vi "MegaAwesome_9_27_12a_JW.vi"() -> ()   [LabVIEW 2011]
uses:
  data/MegaAwesome_States.ctl
  <vilib>/Utility/inputDevices.llb/keyboardAcquire.vi
  <vilib>/Utility/file.llb/Read From Spreadsheet File (string).vi
  <vilib>/Utility/file.llb/Write To Spreadsheet File (string).vi
panel:
  out "Image Center X":i32
  in  "Disable Flag":bool
  out "Index":string
  in  "Slider Min":dbl=5.0
  in  "Slider Max":dbl=5.0
  out "Opj X Axis":string
  out "X Axis Display Type":string
  in  "Index-Sat":dbl=5.0
  in  "Index-Lin":dbl=5.0
  in  "IndexLog-Lin":dbl=5.0
  in  "IndexLog-Sat":dbl=5.0 caption="Num Pts"
  out "Lin Id-Log Used":dbl[](array[numeric])
  out "Lin-Vg Array-Log Used":dbl[](array[numeric])
  in  "New: Comments":string
  out "Save Array":string[][](array[string])
  out "Folder Index":i32 caption="Length"
  out "Sat Id-Used":dbl[](array[numeric])
  out "Sat Vg Array-Used":dbl[](array[numeric])
  out "Vg Array-Log-Used":dbl[](array[numeric])
  out "Sat Id-Log-Used":dbl[](array[numeric])
  out "Lin Id-Used":dbl[](array[numeric])
  out "Lin-Vg Array-Used":dbl[](array[numeric])
  out "Lin Vd":dbl
  out "Recorded Prop":T1
  out "Current State":T2
  in  "Main Tab Control":T3(tab)
  in  "Transfer File":path
  out "Transfer Folder":path
  in  "Transport\nFolder":path caption="Transport Folder"
  out "Transport\nFile":path caption="Transport File"
  in  "Image Folder":path
  out "Image File":path
  out "Fabrication Prop":T4
  out "Distances":i32[](array[numeric])
  in  "Zoom":i32(slide)=-3 scale=-5.0..5.0
  in  "Magnification":i32(ring) items=["5x", "10x", "20x", "50x", "80x"]
  in  "Undo Button":bool
  in  "Remove Button":bool
  in  "Transfer Plots":T5(tab)=enum."Saturation"
  in  "Lin-Trans Slider":dbl(slide) step=1.0 scale=-2.0..2.0 scale format="%#_1p"
  out "Sqrt-Lin":cluster{dbl[], dbl[]}[](graph)
  in  "Sat-Trans Slider":dbl(slide) step=1.0 scale=-2.0..2.0 scale format="%#_1p"
  out "Sqrt-Sat":cluster{dbl[], dbl[]}[](graph)
  out "Raw- Lin":cluster{dbl[], dbl[]}[](graph)
  out "Raw- Sat":cluster{dbl[], dbl[]}[](graph)
  in  "Log Plots":enum32{"Linear", "Saturation", "Transport"}(tab)=enum."Saturation"
  in  "Lin-Log Slider":dbl(slide) step=1.0 scale=-2.0..2.0 scale format="%#_1p"
  out "Lin-Log":cluster{dbl[], dbl[]}[](graph)
  in  "Sat-Log Slider":dbl(slide) step=1.0 scale=-2.0..2.0 scale format="%#_1p"
  out "Sat-Log":cluster{dbl[], dbl[]}[](graph)
  out "Transport":cluster{ext[], ext[]}[](graph)
  out "Transport Name:":string
  in  "Manual Controls":T6
  in  "File Controls":T7
  out "Date Recorded":string="Date Recorded" caption="Measured"
  out "Data Name:":string
  out "Image Name":string
  out "Date Created":string caption="Fabricated"
  in  "Comments:":string
  out "Rec: Length":dbl caption="Length" format="%#_3g"
  out "Rec: Width":dbl caption="Width" format="%#_4g"
  out "Rec: Dielectric (d)":dbl caption="Dielectric (d)" format="%#_3g"
  in  "New: Dielectric":dbl
  in  "New: Length":dbl
  in  "New: Width":dbl
  out "Rec: Temp":dbl caption="Sample Temp" format="%.1f"
  in  "New: Temp":dbl format="%.1f"
  out "Image Out":T8(plugin-control)
  in  "Num Pts":dbl=5.0
  in  "Num Pts Log":dbl=5.0 caption="Num Pts"
  out "Recorded Values Cluster":T9
  out "Calculated Values Cluster":T9 caption="Recorded Values Cluster"
  out "Re-Calculated Values Cluster":T9 caption="Recorded Values Cluster"
  in  "Independant Variable:":string(combo)="Length (um):"
  out "Image Preview":T8(plugin-control)
  out "Total Width":i32
  in  "Index Array":u16(ring) caption="Index" items=["1A", "1A", "1A", "1A", "1A", "1A", "1A", "1A", "1A", "1A", "1A", "1A", "1A", "1A", "1A", "1A", "1A", "1A", "1A", "1A", "1A", "1A", "1A", "1A", "1A", "1A", "1A", "1A", "1A", "1A", "1A", "1A", "1A", "1A", "1A", "1A", "1A"]
  in  "Room Temp":dbl=294.0 caption="Room Temp (K)"
  out "No Image\n File":path=path "\\\\acad1\\physics/Jurchescu-group/JW-PD/Mega Awesome/Image Not Found.png" caption="No Image File"
  out "Origin Project File":path=path "\\\\acad1\\physics/Jurchescu-group/JW-PD/Group Library/Origin Project Files/DeviceData_8_10_12a_JW.opj"
  out "No Transport\n File":path=path "\\\\acad1\\physics/Jurchescu-group/JW-PD/Mega Awesome/No Transport File.txt" caption="No Transport File"
  in  "Transport Style Controls":T10={"Transport Line Size"=1, "Transport Line Color"=16772608} {"Transport Line Size" items=["Extra Small", "Small", "Medium", "Large", "Extra Large"]}
  out "Application Directory":path
  # "1)  Select the Transfer File that you would like to analyze:"
  # "Transfer Location"
  # "2) What else would you like to view during your analysis?"
  # "Transport Location"
  # "Image Location"
  # "Recorded"
  # "Calculated"
  # "Re-Calculated"
  # "Manual"
  # "um"
  # "Slider\nDoesn't\nWork"
  # "V"
  # "V"
  # "Slider\nDoesn't\nWork"
  # "V"
  # "Default File Choices"
  # "Default Analysis Values"
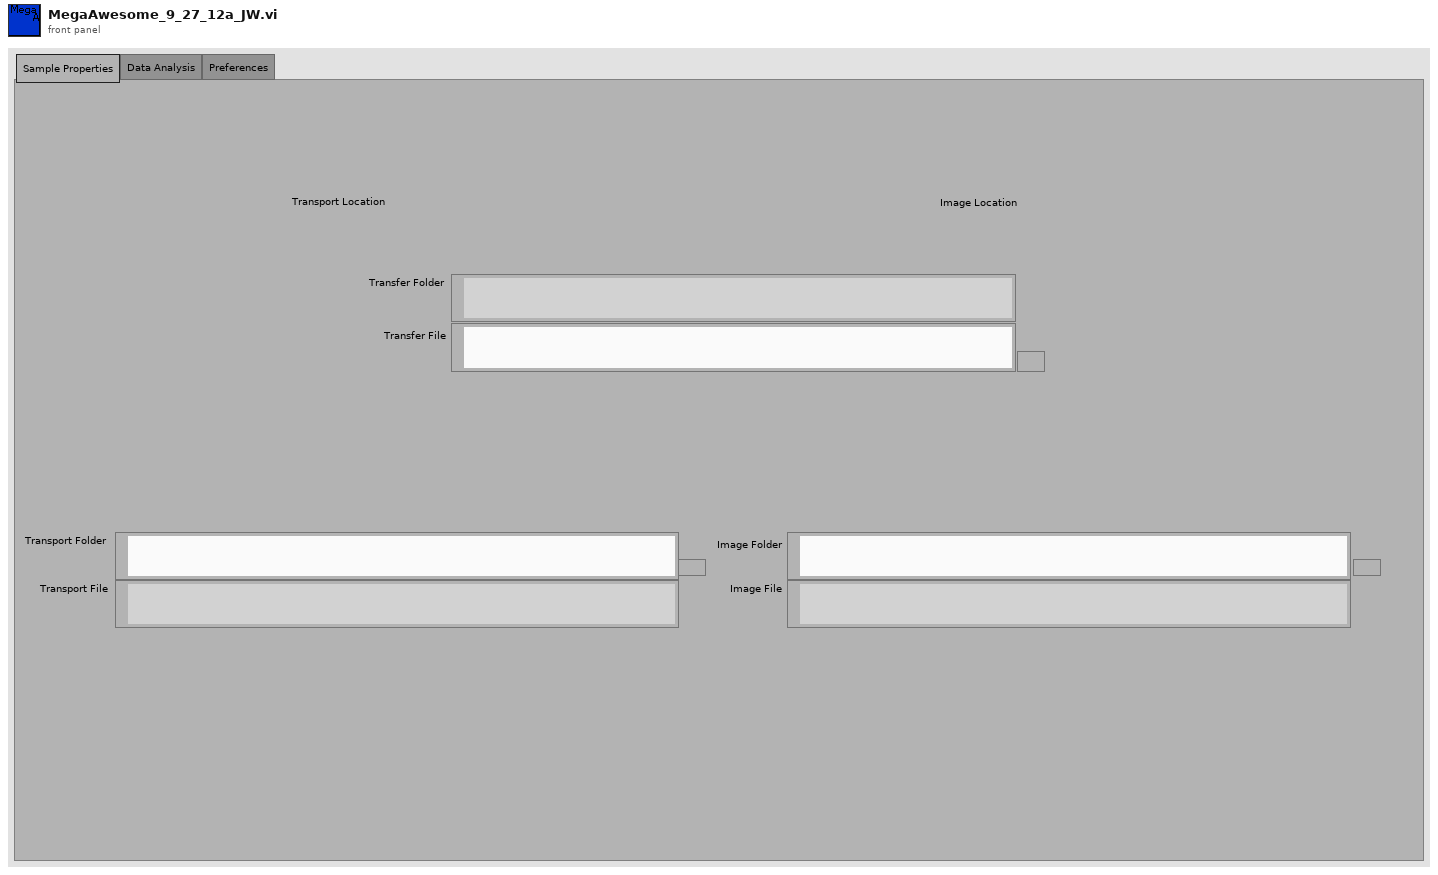
[diagram p1: front panel]
types:
  T1 = cluster{"Date Recorded":string, "Index":string, "Length":dbl, "Width":dbl, "Sample Temp":dbl}
  T2 = typedef "MegaAwesome_States.ctl" = enum16{"Init", "File Missing", "No Event", "Read Data", "Calculated Values", "Re-Calculated Values", "Next File", "Previous File", "Discard File", "Save", "Save Lines", "Export", "Exit"}
  T3 = enum32{"Sample Properties", "Data Analysis", "Preferences"}
  T4 = cluster{"Date Created":string, "Material":string, "Solvent":string, "Concentration":dbl, "Method":string, "Dielectric (nm)":dbl, "Treatment":string, "Comments":string}
  T5 = enum32{"Linear", "Saturation", "Raw-Linear", "Raw-Saturation"}
  T6 = cluster{"Manual-Temp":bool, "Manual-Width":bool, "Manuel-Length":bool, "Manuel-Dielectric":bool, "Manual Comments":bool}
  T7 = cluster{"Previous File":bool, "Discard ":bool, "Save Lines":bool, "Close":bool, "Next File ":bool, "Save":bool, "Save Next":bool, "Export":bool}
  T8 = typedef "IMAQ Image.ctl" = refnum<image>
  T9 = cluster{"Mobility-Sat":dbl, "Moblitity-Lin":dbl, "On/Off":dbl, "Off Current":dbl, "Vt-Sat":dbl, "STS":dbl, "Trap Density-VT":dbl, "Trap Density-STS":dbl}
  T10 = cluster{"Transport Line Size":u16, "Transport Line Color":u32}
  T11 = typedef "LVBoundsTypeDef.ctl" = cluster{"Width":u32, "Height":u32}
  T12 = enum16{"0", "1", "2", "3", "4", "5", "6", "7", "8", "9", "A", "B", "C", "D", "E", "F", "G", "H", "I", "J", "K", "L", "M", "N", "O", "P", "Q", "R", "S", "T", "U", "V", "W", "X", "Y", "Z", "F1", "F2", "F3", "F4", "F5", "F6", "F7", "F8", "F9", "F10", "F11", "F12", "F13", "F14", "F15", "ADD", "BACK", "BACKSLASH", "CAPITAL", "COMMA", "DECIMAL", "DELETE", "DIVIDE", "DOWN", "END", "EQUALS", "ESCAPE", "GRAVE (`)", "HOME", "INSERT", "LBRACKET", "LCONTROL", "LEFT", "L ALT", "LSHIFT", "LWIN", "MINUS", "MULTIPLY", "NEXT", "NUMLOCK", "NUMPAD_0", "NUMPAD_1", "NUMPAD_2", "NUMPAD_3", "NUMPAD_4", "NUMPAD_5", "NUMPAD_6", "NUMPAD_7", "NUMPAD_8", "NUMPAD_9", "PAUSE", "PERIOD", "PRIOR (PG UP)", "RBRACKET", "RCONTROL", "RETURN", "RIGHT", "R ALT", "RSHIFT", "RWIN", "SCROLL", "SEMICOLON", "SLASH", "SPACE", "SUBTRACT", "TAB", "UP", "ENTER (num pad)", "' (quote)"}[]
  T13 = enum16{"0", "1", "2", "3", "4", "5", "6", "7", "8", "9", "A", "B", "C", "D", "E", "F", "G", "H", "I", "J", "K", "L", "M", "N", "O", "P", "Q", "R", "S", "T", "U", "V", "W", "X", "Y", "Z", "F1", "F2", "F3", "F4", "F5", "F6", "F7", "F8", "F9", "F10", "F11", "F12", "F13", "F14", "F15", "ADD", "BACK", "BACKSLASH", "CAPITAL", "COMMA", "DECIMAL", "DELETE", "DIVIDE", "DOWN", "END", "EQUALS", "ESCAPE", "GRAVE (`)", "HOME", "INSERT", "LBRACKET", "LCONTROL", "LEFT", "L ALT", "LSHIFT", "LWIN", "MINUS", "MULTIPLY", "NEXT", "NUMLOCK", "NUMPAD_0", "NUMPAD_1", "NUMPAD_2", "NUMPAD_3", "NUMPAD_4", "NUMPAD_5", "NUMPAD_6", "NUMPAD_7", "NUMPAD_8", "NUMPAD_9", "PAUSE", "PERIOD", "PRIOR (PG UP)", "RBRACKET", "RCONTROL", "RETURN", "RIGHT", "R ALT", "RSHIFT", "RWIN", "SCROLL", "SEMICOLON", "SLASH", "SPACE", "SUBTRACT", "TAB", "UP", "ENTER (num pad)", "' (quote)"}
  T14 = typedef "ROI Descriptor" = cluster{"Global Rectangle":i32[], "Contours":cluster{"ID":enum32{"External", "Internal"}, "Type":u32, "Coordinates":i32[]}[]}
  T15 = cluster{string, sgl, bool, bool, bool, bool, bool, bool, i32}
  T16 = cluster{i32, cluster{string, sgl, bool, bool, bool, bool, bool, bool, i32}, i32, i32}
  T17 = cluster{"Global Rectangle":i32[], "Contours":cluster{"Contour Type":u32, "ROI Type":u32, "Points":i32[]}[]}
  T18 = cluster{"Contour Type":u32, "ROI Type":u32, "Points":i32[]}[]
  T19 = cluster{"[0]":cluster{dbl[], dbl[]}, "[1]":cluster{dbl[], dbl[]}, "[2]":cluster{dbl[], dbl[]}, "[3]":cluster{dbl[], dbl[]}, "[4]":cluster{dbl[], dbl[]}, "[5]":cluster{dbl[], dbl[]}, "[6]":cluster{dbl[], dbl[]}, "[7]":cluster{dbl[], dbl[]}, "[8]":cluster{dbl[], dbl[]}}
  T20 = cluster{i32[], cluster{"Contour Type":u32, "ROI Type":u32, "Points":i32[]}[]}
  T21 = cluster{"Contour Type":u32, "ROI Type":u32, "Points":i32[]}
  T22 = cluster{"Points[0]":i32, "Points[1]":i32, "Points[2]":i32, "Points[3]":i32, "Points[4]":i32, "Points[5]":i32, "Points[6]":i32, "Points[7]":i32, "Points[8]":i32}
  T23 = cluster{"Sat Vg Used":dbl[], "Sat Sqrt(Id) Used ":dbl[], "Lin Vg Used":dbl[], "Lin Sqrt(Id) Used":dbl[], "Index-Lin":dbl, "Index-Sat":dbl}
  T24 = cluster{"Raw Sat":cluster{dbl[], dbl[]}[], "Sqrt Sat":cluster{dbl[], dbl[]}[], "Log Sat":cluster{dbl[], dbl[]}[], "Raw Lin":cluster{dbl[], dbl[]}[], "Sqrt Lin":cluster{dbl[], dbl[]}[], "Log Lin":cluster{dbl[], dbl[]}[]}
  T25 = cluster{"Mobility-Sat":dbl, "Vt-Sat":dbl, "Mobility-Lin":dbl, "Vt-Lin":dbl, "Off I-Sat":dbl, "On/Off I-Sat":dbl}
  T26 = cluster{"Sat Vg Used":dbl[], "Sat Log(Id) Used":dbl[], "Lin Vg Used":dbl[], "Lin Log(Id) Used":dbl[], "STS Index-Sat":dbl, "STS Index-Lin":dbl}
  T27 = cluster{"Independant  Variable Indicator":string, "Parameter String Indicator":string}
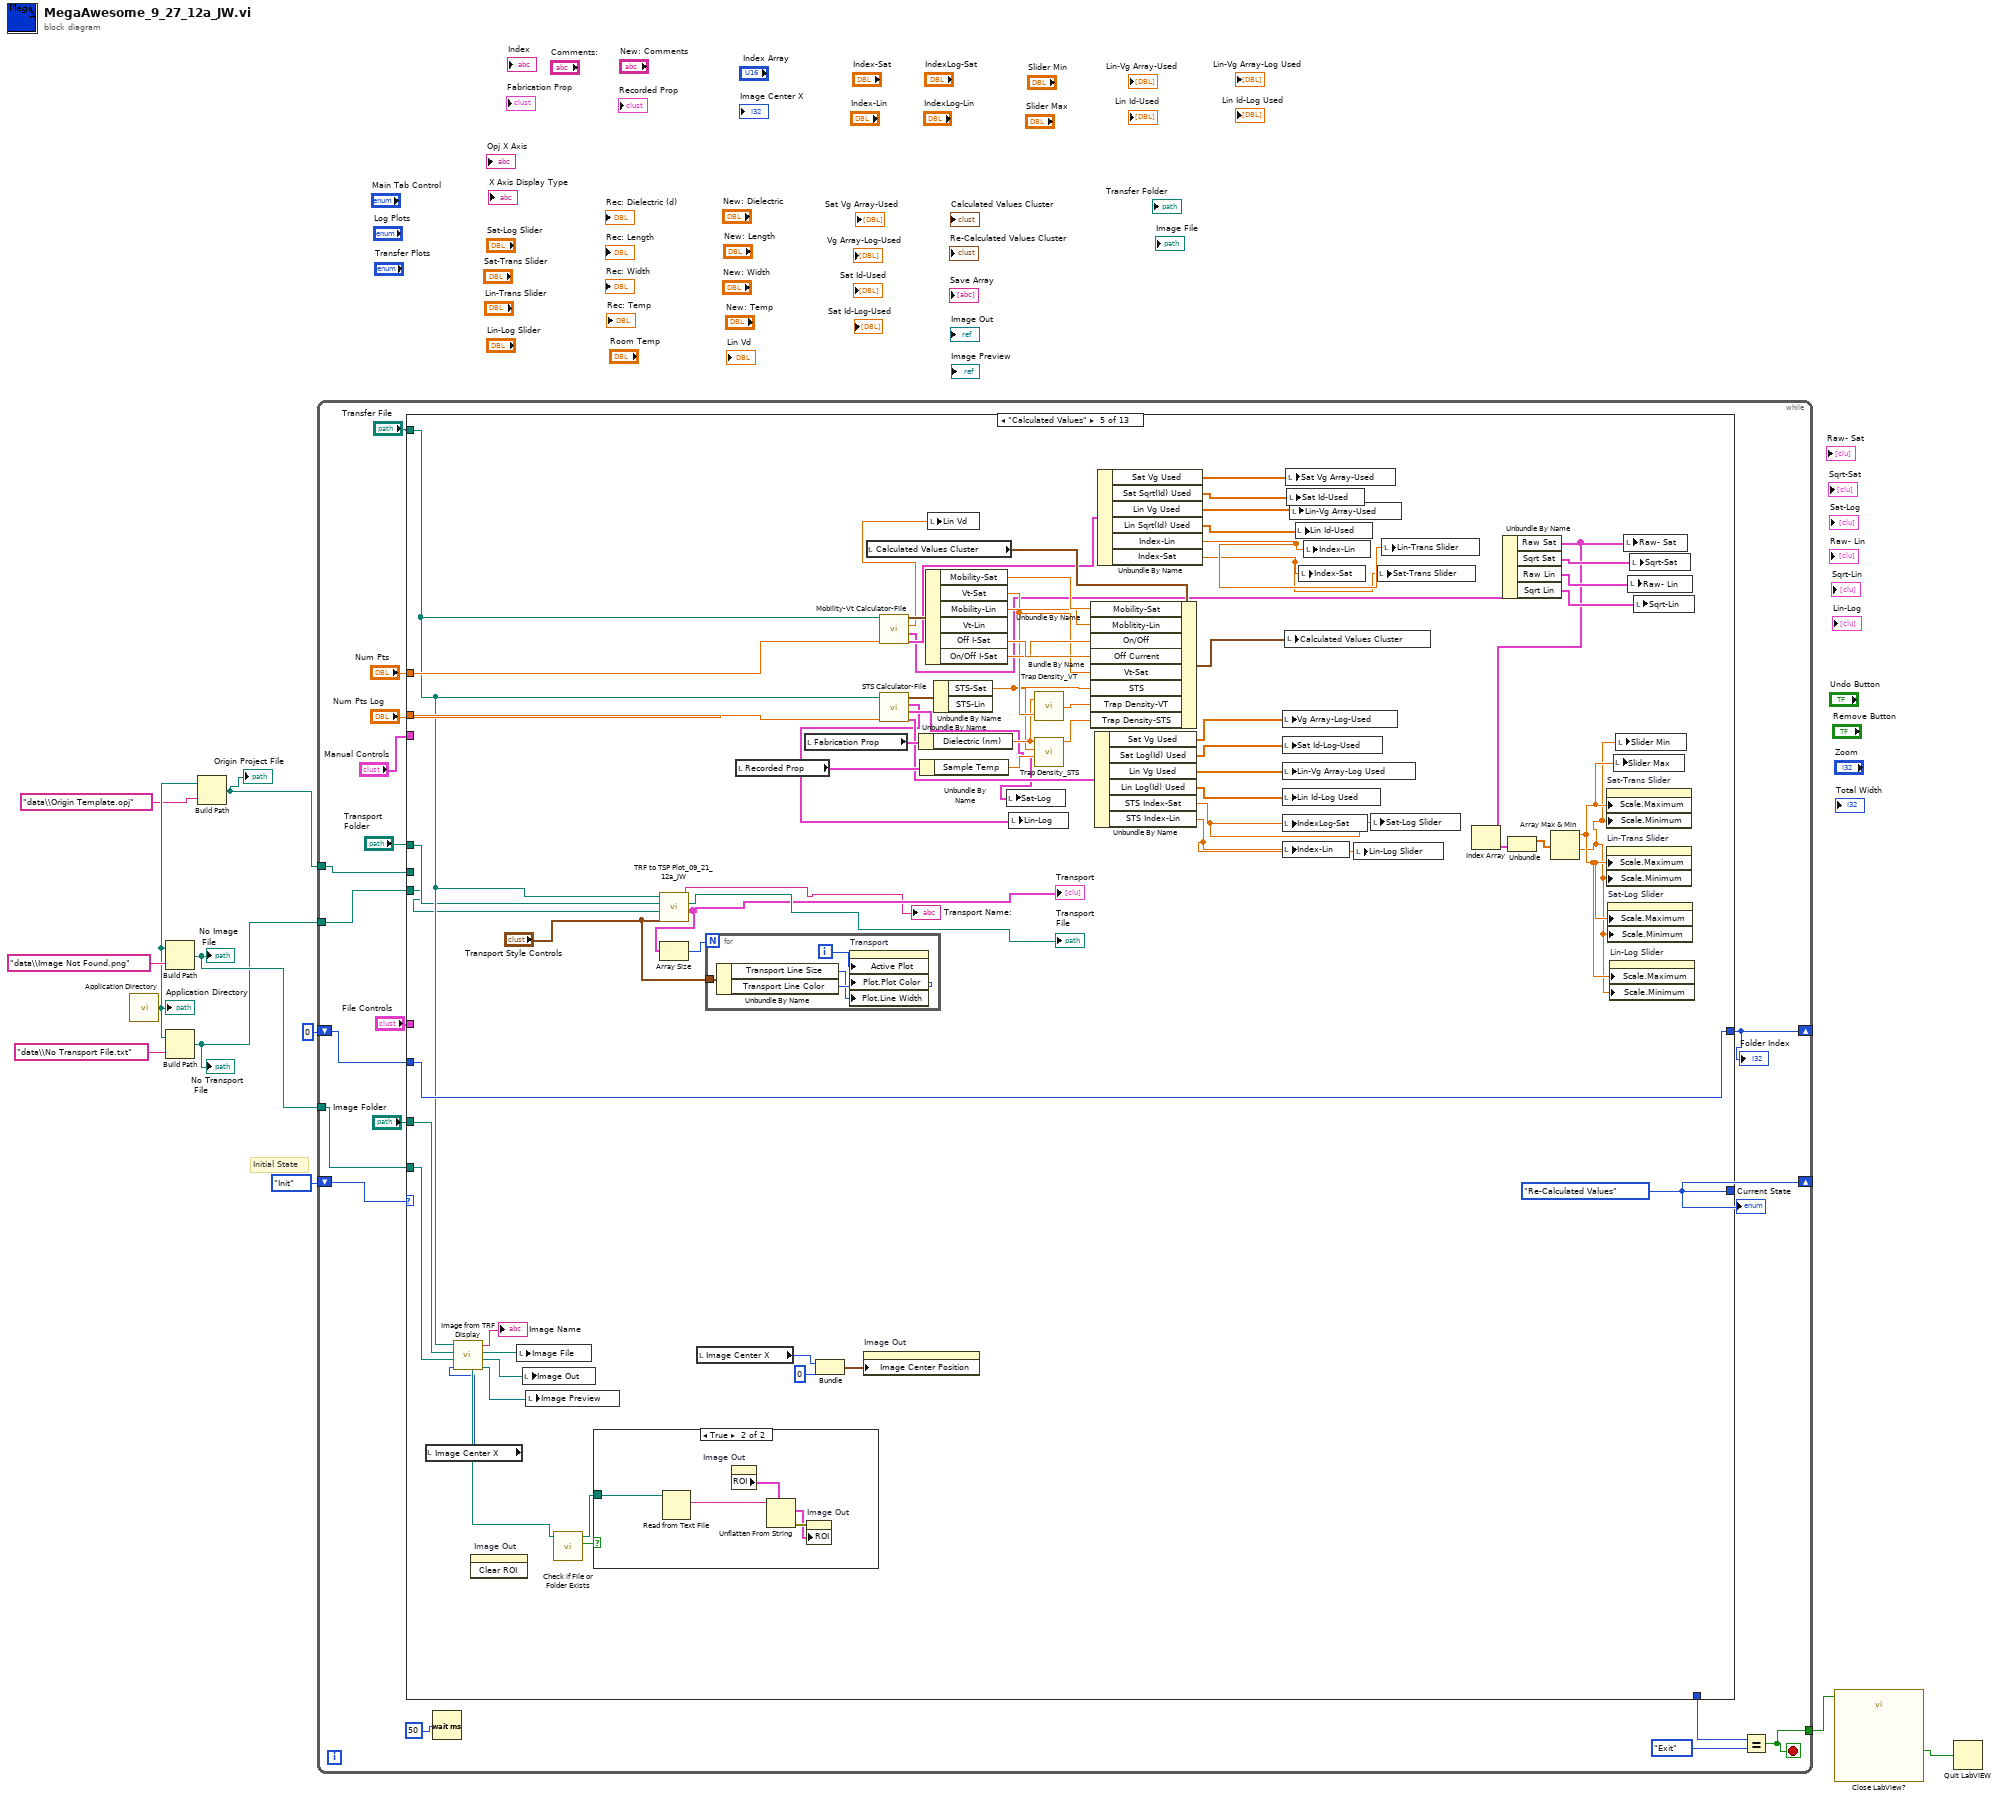
[diagram p0: block diagram]
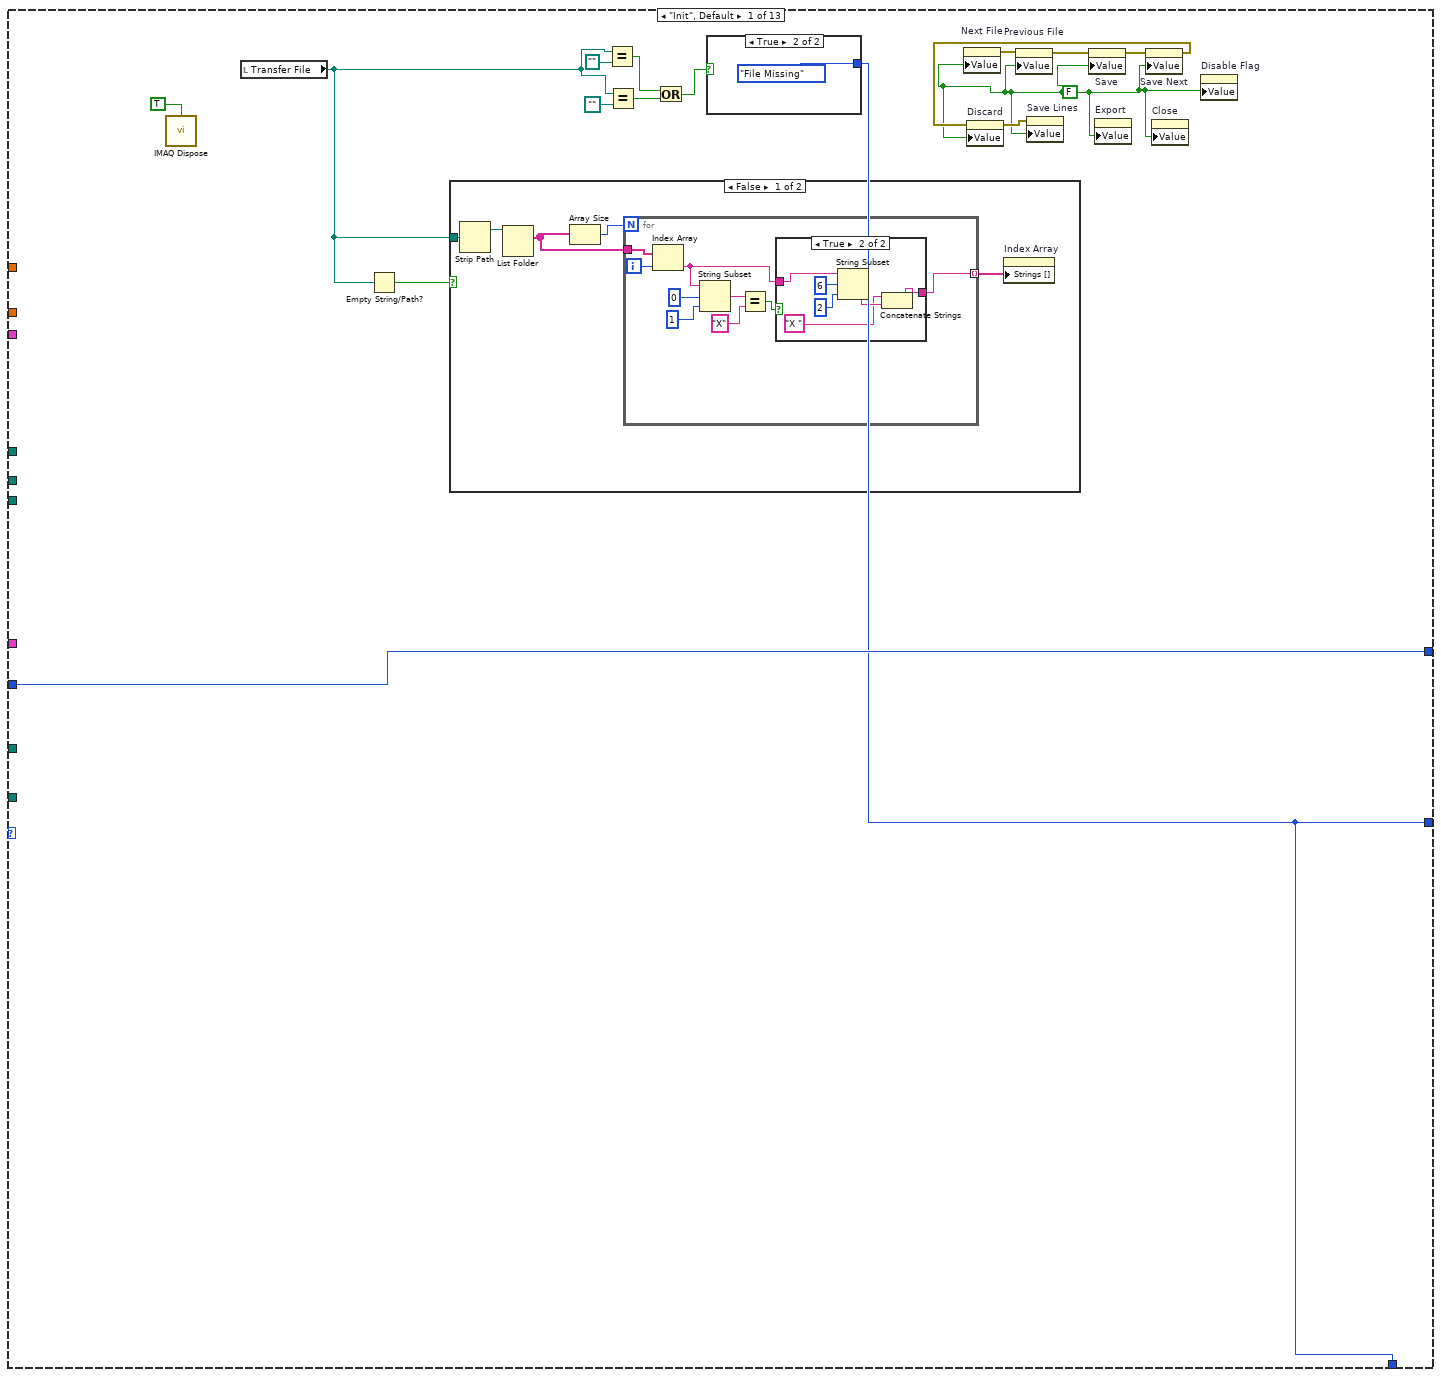
[diagram p2: hidden frame]
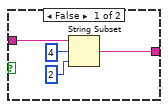
[diagram p3: hidden frame]
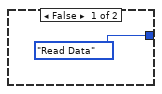
[diagram p5: hidden frame]
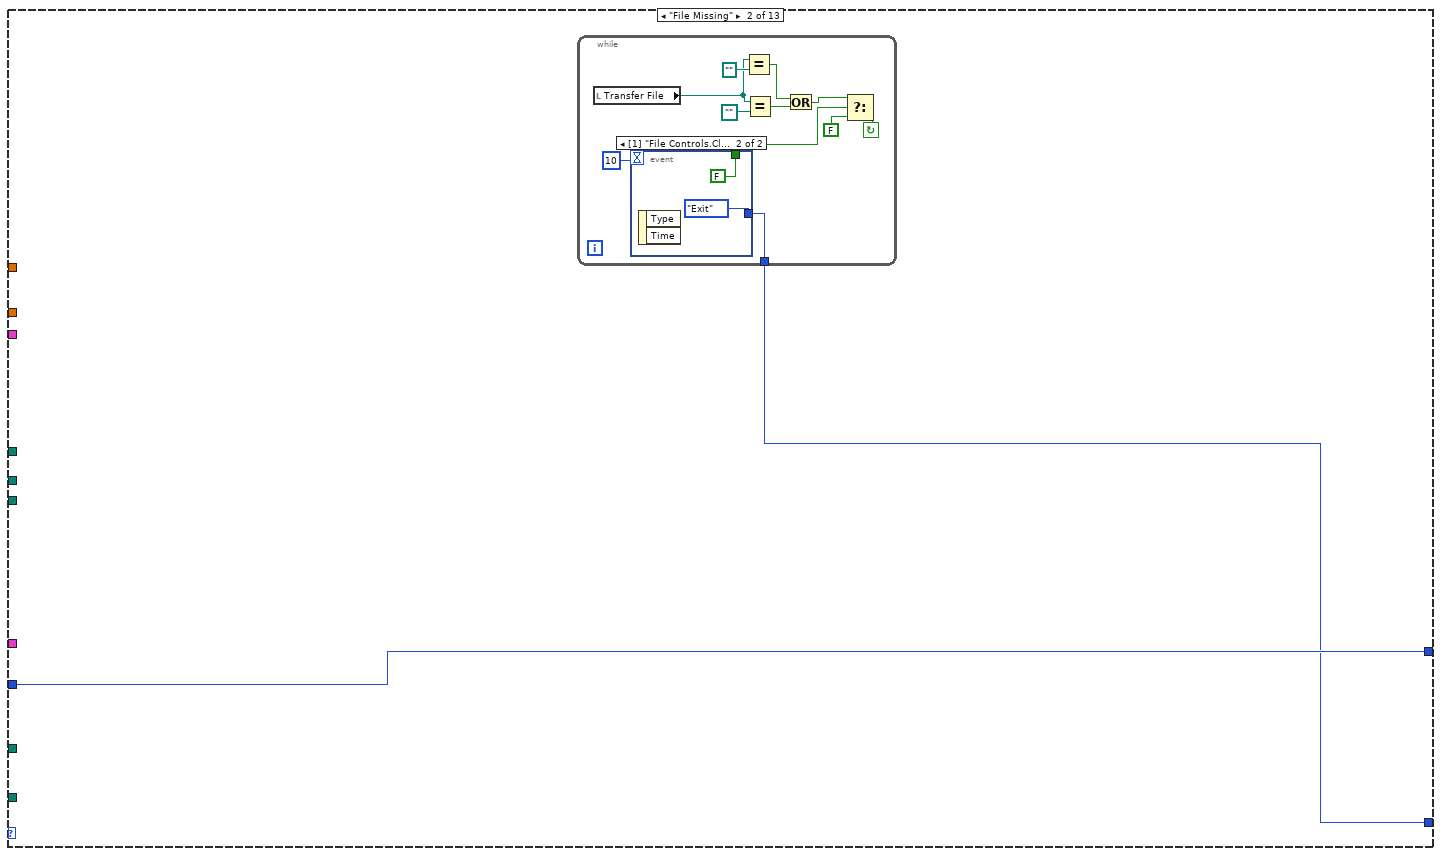
[diagram p6: hidden frame]
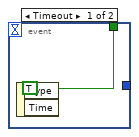
[diagram p7: hidden frame]
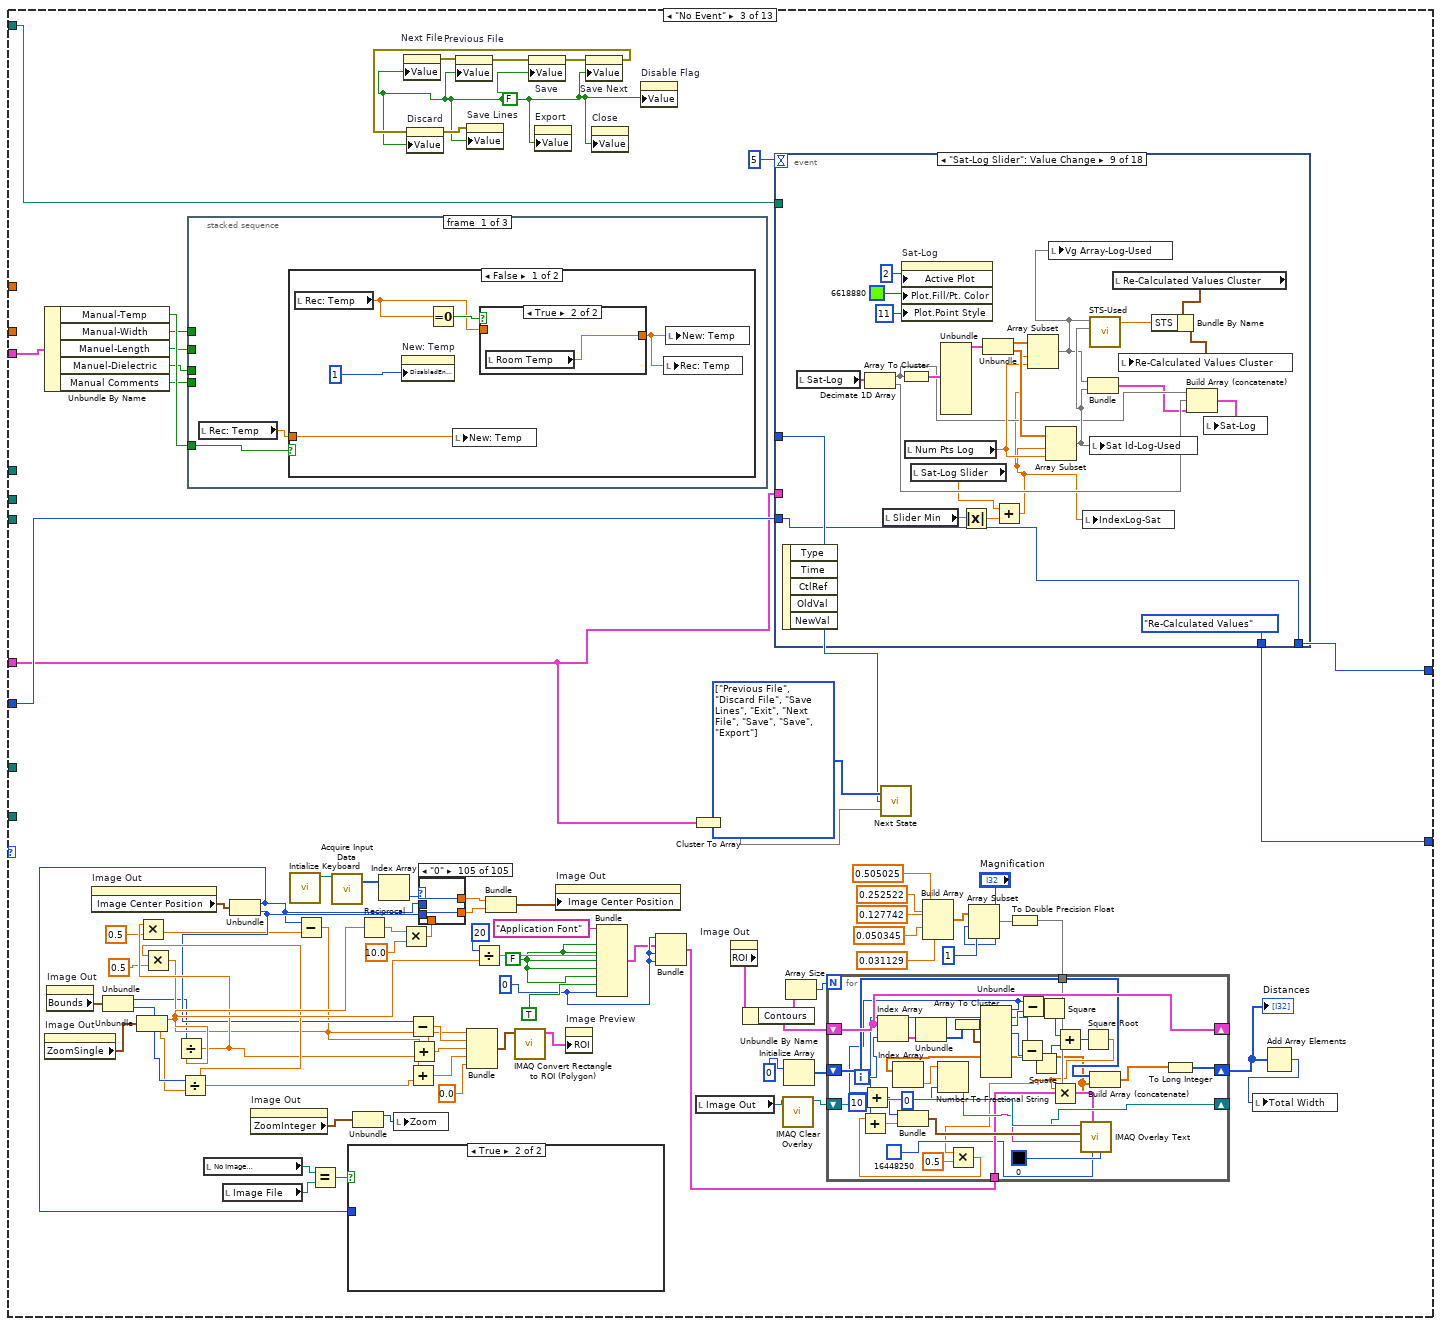
[diagram p8: hidden frame]
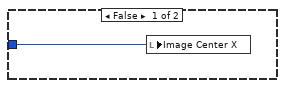
[diagram p9: hidden frame]
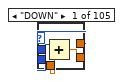
[diagram p10: hidden frame]
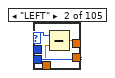
[diagram p11: hidden frame]
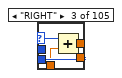
[diagram p12: hidden frame]
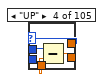
[diagram p13: hidden frame]
diagram:
  # "Initial State"
  n1 = call <vilib>:"Application Directory.vi"() -> ("Application Directory"=w4:path)
  "Application Directory" <- w4
  n2 = Build Path(base path=w4, name or relative path="data\\Image Not Found.png") -> (appended path=w7:path)
  "No Image\n File" <- w7
  n3 = Build Path(base path=w4, name or relative path="data\\No Transport File.txt") -> (appended path=w6:path)
  "No Transport\n File" <- w6
  n4 = Build Path(base path=w4, name or relative path="data\\Origin Template.opj") -> (appended path=w5:path)
  "Origin Project File" <- w5
  n5 = while {
    shift-right: [w16] -> _
    shift-left: MegaAwesome_States."Init" -> [w14]
    shift-right: [w23] -> _
    shift-left: 0 -> [w24]
    tunnel: w7 -> [w20]
    tunnel: w6 -> [w18]
    tunnel: w5 -> [w17]
    tunnel: [w15] -> w2
    stop <- w15 stop-if-true
    n6 = case shown="\"Calculated Values\"" w14 {
      tunnel: [w30 w72 w162 MegaAwesome_States."Calculated Values" MegaAwesome_States."Re-Calculated Values" MegaAwesome_States."No Event" MegaAwesome_States."Read Data" MegaAwesome_States."Read Data" MegaAwesome_States."Init" w814 w1335 MegaAwesome_States."No Event" MegaAwesome_States."Exit"] -> w16
      tunnel: "Transfer File" -> [_ _ w153 w606 w654 _ w755 w766 w784 w819 _ _ _]
      tunnel: "Num Pts" -> [_ _ _ _ w689 _ _ _ _ _ _ _ _]
      tunnel: "Num Pts Log" -> [_ _ _ _ w688 _ _ _ _ _ _ _ _]
      tunnel: "Image Folder" -> [_ _ _ _ w685 _ _ _ _ _ _ w1346 _]
      tunnel: w20 -> [_ _ _ _ w684 _ _ _ _ _ _ _ _]
      tunnel: [w40 w73 w154 w611 w683 w715 w741 w764 w779 w820 w1336 w1356 w1362] -> w23
      tunnel: w24 -> [w40 w73 w155 w609 w683 w715 w742 w765 _ w820 w1336 w1356 w1362]
      tunnel: "Manual Controls" -> [_ _ w164 _ _ _ _ _ _ w818 _ _ _]
      tunnel: "File Controls" -> [_ _ w151 _ _ _ _ _ _ w813 _ _ _]
      tunnel: "Transport\nFolder" -> [_ _ _ _ w650 _ _ _ _ _ _ _ _]
      tunnel: w18 -> [_ _ _ _ w649 _ _ _ _ _ _ _ _]
      tunnel: w17 -> [_ _ _ _ _ _ _ _ _ _ _ _ w1361]
      tunnel: [w30 _ _ _ _ _ _ _ _ _ w1334 _ _] -> w13
      frame "Init", Default {
        w31 = FALSE
        n7 = call "IMAQ Dispose"("All Images? (No)"=TRUE) -> ()  [unwired: 5 in, 1 out]
        n8 = local read "Transfer File"() -> (w38:path)
        n9 = Empty String/Path?(string/path=w38) -> (empty?=w39:bool)
        n10 = case shown="False" w39 {
          tunnel: w38 -> [w47 _]
          frame False {
            n11 = Strip Path(path=w47) -> (stripped path=w49:path)  [unwired: 1 out]
            n12 = List Folder(path=w49) -> (filenames=w48:string[])  [unwired: 3 in, 3 out]
            n13 = Array Size(array=w48) -> (size(s)=w50:i32)
            n14 = for {
              N: w50 -> [_]
              tunnel: w48 -> [w59]
              tunnel: [w57] -> w46 mode=indexing
              i -> [w58]
              n15 = Index Array(array=w59, index=w58) -> (element=w56:string)
              n16 = String Subset(string=w56, offset (0)=0, length (rest)=1) -> (substring=w53:string)
              n17 = Equal?(x=w53, y="X") -> (x = y?=w52:bool)
              n18 = case shown="True" w52 {
                tunnel: w56 -> [w63 w67]
                tunnel: [w60 w66] -> w57
                frame False {
                  n19 = String Subset(string=w63, offset (0)=4, length (rest)=2) -> (substring=w60:string)
                }
                frame True {
                  n20 = String Subset(string=w67, offset (0)=6, length (rest)=2) -> (substring=w65:string)
                  n21 = Concatenate Strings("X ", w65) -> (w66:string)
                }
              }
            }
            n22 = property on="Index Array" class="Ring (strict)"("Strings []"=w46) -> ()  [unwired: 2 in, 2 out]
          }
          frame True {
          }
        }
        n23 = Equal?(x=w38, y=path "") -> (x = y?=w43:bool)
        n24 = Equal?(x=w38, y=path "") -> (x = y?=w42:bool)
        n25 = Or(x=w43, y=w42) -> (x .or. y?=w45:bool)
        n26 = case shown="True" w45 {
          tunnel: [MegaAwesome_States."Read Data" MegaAwesome_States."File Missing"] -> w30
          frame False {
          }
          frame True {
          }
        }
        n27 = property on="Next File" class="Bool (strict)"("Value"=w31) -> (error out=w36:errorcluster)  [unwired: 2 in, 1 out]
        n28 = property on="Previous File" class="Bool (strict)"(error in=w36, "Value"=w31) -> (error out=w35:errorcluster)  [unwired: 1 in, 1 out]
        n29 = property on="Save" class="Bool (strict)"(error in=w35, "Value"=w31) -> (error out=w34:errorcluster)  [unwired: 1 in, 1 out]
        n30 = property on="Export" class="Bool (strict)"("Value"=w31) -> ()  [unwired: 2 in, 2 out]
        n31 = property on="Save Next" class="Bool (strict)"(error in=w34, "Value"=w31) -> (error out=w33:errorcluster)  [unwired: 1 in, 1 out]
        n32 = property on="Discard" class="Bool (strict)"(error in=w33, "Value"=w31) -> (error out=w32:errorcluster)  [unwired: 1 in, 1 out]
        n33 = property on="Save Lines" class="Bool (strict)"(error in=w32, "Value"=w31) -> ()  [unwired: 1 in, 2 out]
        n34 = property on="Close" class="Bool (strict)"("Value"=w31) -> ()  [unwired: 2 in, 2 out]
        n35 = property on="Disable Flag" class="Bool (strict)"("Value"=w31) -> ()  [unwired: 2 in, 2 out]
      }
      frame "File Missing" {
        n36 = while {
          tunnel: [w79] -> w72
          stop <- w75 continue-if-true
          n37 = local read "Transfer File"() -> (w80:path)
          n38 = event shown="[1] \"File Controls.Close\": Value Change" {
            selector: _ -> [_ _]
            dyn-events: _ -> [_ _]
            timeout: 10 -> [_ _]
            tunnel: [_ MegaAwesome_States."Exit"] -> w79
            tunnel: [TRUE FALSE] -> w78
            event Timeout {
              n39 = event-data() -> ()  [unwired: 1 in, 2 out]
            }
            event "File Controls.Close": Value Change {
              n40 = event-data() -> ()  [unwired: 1 in, 2 out]
            }
          }
          n41 = Equal?(x=w80, y=path "") -> (x = y?=w82:bool)
          n42 = Equal?(x=w80, y=path "") -> (x = y?=w83:bool)
          n43 = Or(x=w82, y=w83) -> (x .or. y?=w77:bool)
          n44 = Select(t=w77, s=w78, f=FALSE) -> (s? t:f=w75:bool)
        }
      }
      frame "No Event" {
        w142 = FALSE
        w144 = 0
        w152 = FALSE
        w171 = T2[] [enum."Previous File", enum."Discard File", enum."Save Lines", enum."Exit", enum."Next File", enum."Save", enum."Save", enum."Export"] items=["Init", "File Missing", "No Event", "Read Data", "Calculated Values", "Re-Calculated Values", "Next File", "Previous File", "Discard File", "Save", "Save Lines", "Export", "Exit"]
        n45 = Unbundle By Name(w164) -> ("Manual-Temp"=w169:bool, "Manual-Width"=w168:bool, "Manuel-Length"=w167:bool, "Manuel-Dielectric"=w166:bool, "Manual Comments"=w165:bool)
        n46 = property on="Image Out" class="ImageControl"() -> ("ZoomSingle"=w128:cluster{"X":sgl, "Y":sgl})  [unwired: 2 in, 2 out]
        n47 = property on="Image Out" class="ImageControl"() -> ("Bounds"=w127:T11)  [unwired: 2 in, 2 out]
        n48 = property on="Image Out" class="ImageControl"() -> ("Image Center Position"=w121:cluster{"X":u32, "Y":u32})  [unwired: 2 in, 2 out]
        n49 = Unbundle(w127) -> ("Width"=w130:u32, "Height"=w131:u32)
        n50 = Unbundle(w128) -> ("X"=w148:sgl, "Y"=w129:sgl)
        n51 = Divide(x=w130, y=w148) -> (x/y=w139:sgl)
        n52 = Multiply(x=w139, y=0.5) -> (x*y=w134:dbl)
        n53 = Divide(x=w131, y=w129) -> (x/y=w140:sgl)
        n54 = Multiply(x=w140, y=0.5) -> (x*y=w135:dbl)
        n55 = stacked-sequence {
          tunnel: w169 -> [w565 _ _]
          tunnel: w168 -> [_ w574 _]
          tunnel: w167 -> [_ _ w590]
          tunnel: w166 -> [_ _ w587]
          tunnel: w165 -> [_ _ w586]
          frame #0 {
            n56 = local read "Rec: Temp"() -> (w564:dbl)
            n57 = case shown="False" w565 {
              tunnel: w564 -> [w570 _]
              frame False {
                n58 = local read "Rec: Temp"() -> (w568:dbl)
                n59 = property on="New: Temp" class="DigNum (strict)"("DisabledEnum"=1) -> ()  [unwired: 2 in, 2 out]
                n60 = Equal To 0?(x=w568) -> (x = 0?=w569:bool)
                n61 = local write "New: Temp"(w570) -> ()
                n62 = case shown="True" w569 {
                  tunnel: [w571 w572] -> w566
                  tunnel: w568 -> [w571 _]
                  frame False {
                  }
                  frame True {
                    n63 = local read "Room Temp"() -> (w572:dbl)
                  }
                }
                n64 = local write "Rec: Temp"(w566) -> ()
                n65 = local write "New: Temp"(w566) -> ()
              }
              frame True {
                n66 = property on="New: Temp" class="DigNum (strict)"("DisabledEnum"=0) -> ()  [unwired: 2 in, 2 out]
              }
            }
          }
          frame #1 {
            n67 = case shown="True" w574 {
              frame False {
                n68 = property on="New: Width" class="DigNum (strict)"("DisabledEnum"=1) -> ()  [unwired: 2 in, 2 out]
              }
              frame True {
                n69 = property on="New: Width" class="DigNum (strict)"("DisabledEnum"=0) -> ()  [unwired: 2 in, 2 out]
              }
            }
            n70 = local read "Total Width"() -> (w580:i32)
            n71 = Equal To 0?(x=w580) -> (x = 0?=w577:bool)
            n72 = local read "Rec: Width"() -> (w578:dbl)
            n73 = Not(x=w574) -> (.not. x?=w576:bool)
            n74 = Or(x=w577, y=w574) -> (x .or. y?=w579:bool)
            n75 = And(x=w577, y=w576) -> (x .and. y?=w575:bool)
            n76 = case shown="True" w575 {
              tunnel: w578 -> [_ w583]
              frame False {
              }
              frame True {
                n77 = local write "New: Width"(w583) -> ()
              }
            }
            n78 = case shown="True" w579 {
              tunnel: w580 -> [w584 _]
              frame False {
                n79 = local write "New: Width"(w584) -> ()
              }
              frame True {
                n80 = property on="New: Width" class="DigNum (strict)"("DisabledEnum"=0) -> ()  [unwired: 2 in, 2 out]
              }
            }
          }
          frame #2 {
            n81 = local read "Rec: Length"() -> (w591:dbl)
            n82 = case shown="False" w590 {
              tunnel: w591 -> [w599 _]
              frame False {
                n83 = local write "New: Length"(w599) -> ()
                n84 = property on="New: Length" class="DigNum (strict)"("DisabledEnum"=1) -> ()  [unwired: 2 in, 2 out]
              }
              frame True {
                n85 = property on="New: Length" class="DigNum (strict)"("DisabledEnum"=0) -> ()  [unwired: 2 in, 2 out]
              }
            }
            n86 = local read "Comments:"() -> (w588:string)
            n87 = local read "Rec: Dielectric (d)"() -> (w589:dbl)
            n88 = case shown="False" w586 {
              tunnel: w588 -> [w593 _]
              frame False {
                n89 = local write "New: Comments"(w593) -> ()
                n90 = property on="New: Comments" class="Str"("DisabledEnum"=1) -> ()  [unwired: 2 in, 2 out]
              }
              frame True {
                n91 = property on="New: Comments" class="Str"("DisabledEnum"=0) -> ()  [unwired: 2 in, 2 out]
              }
            }
            n92 = case shown="False" w587 {
              tunnel: w589 -> [w596 _]
              frame False {
                n93 = local write "New: Dielectric"(w596) -> ()
                n94 = property on="New: Dielectric" class="DigNum (strict)"("DisabledEnum"=1) -> ()  [unwired: 2 in, 2 out]
              }
              frame True {
                n95 = property on="New: Dielectric" class="DigNum (strict)"("DisabledEnum"=0) -> ()  [unwired: 2 in, 2 out]
              }
            }
          }
        }
        n96 = local read "No Image\n File"() -> (w92:path)
        n97 = local read "Image File"() -> (w91:path)
        n98 = Unbundle(w121) -> ("X"=w93:u32, "Y"=w138:u32)
        n99 = property on="Image Out" class="ImageControl"() -> ("ZoomInteger"=w96:cluster{"X":i32, "Y":i32})  [unwired: 2 in, 2 out]
        n100 = call <vilib>:"Intialize Keyboard.vi"() -> ("device ID"=w118:refnum<k1>)  [unwired: 10 in, 1 out]
        n101 = Subtract(x=w93, y=w134) -> (x-y=w136:dbl)
        n102 = Equal?(x=w92, y=w91) -> (x = y?=w90:bool)
        n103 = call-poly <vilib>:"Acquire Input Data.vi"("device ID"=w118) -> ("keys pressed"=w119:T12)  [unwired: 16 in, 2 out]
        n104 = case shown="True" w90 {
          tunnel: w93 -> [w172 _]
          frame False {
            n105 = local write "Image Center X"(w172) -> ()
          }
          frame True {
          }
        }
        n106 = Unbundle(w96) -> ("X"=w95:i32)  [unwired: 1 out]
        n107 = Reciprocal(x=w148) -> (1/x=w149:sgl)
        n108 = Index Array(array=w119) -> (element=w115:T13)  [unwired: 1 in]
        n109 = local write "Zoom"(w95) -> ()
        n110 = Multiply(x=w149, y=sgl 10.0) -> (x*y=w147:sgl)
        n111 = property on="Next File" class="Bool (strict)"("Value"=w152) -> (error out=w160:errorcluster)  [unwired: 2 in, 1 out]
        n112 = Subtract(x=w138, y=w135) -> (x-y=w137:dbl)
        n113 = Add(x=w137, y=w140) -> (x+y=w123:dbl)
        n114 = Add(x=w136, y=w139) -> (x+y=w122:dbl)
        n115 = case shown="\"0\"" w115 {
          tunnel: w93 -> [w208 w214 w218 w220 w224 w226 w228 w230 w232 w234 w236 w238 w240 w242 w244 w246 w248 w250 w252 w254 w256 w258 w260 w262 w264 w266 w268 w270 w272 w274 w276 w278 w280 w282 w284 w286 w288 w290 w292 w294 w296 w298 w300 w302 w304 w306 w308 w310 w312 w314 w316 w318 w320 w322 w324 w326 w328 w330 w332 w334 w336 w338 w340 w342 w344 w346 w348 w350 w352 w354 w356 w358 w360 w362 w364 w366 w368 w370 w372 w374 w376 w378 w380 w382 w384 w386 w388 w390 w392 w394 w396 w398 w400 w402 w404 w406 w408 w410 w412 w414 w416 w418 w420 w422 w424]
          tunnel: [w208 w213 w217 w220 w224 w226 w228 w230 w232 w234 w236 w238 w240 w242 w244 w246 w248 w250 w252 w254 w256 w258 w260 w262 w264 w266 w268 w270 w272 w274 w276 w278 w280 w282 w284 w286 w288 w290 w292 w294 w296 w298 w300 w302 w304 w306 w308 w310 w312 w314 w316 w318 w320 w322 w324 w326 w328 w330 w332 w334 w336 w338 w340 w342 w344 w346 w348 w350 w352 w354 w356 w358 w360 w362 w364 w366 w368 w370 w372 w374 w376 w378 w380 w382 w384 w386 w388 w390 w392 w394 w396 w398 w400 w402 w404 w406 w408 w410 w412 w414 w416 w418 w420 w422 w424] -> w116
          tunnel: w138 -> [w210 w212 w216 w222 w223 w225 w227 w229 w231 w233 w235 w237 w239 w241 w243 w245 w247 w249 w251 w253 w255 w257 w259 w261 w263 w265 w267 w269 w271 w273 w275 w277 w279 w281 w283 w285 w287 w289 w291 w293 w295 w297 w299 w301 w303 w305 w307 w309 w311 w313 w315 w317 w319 w321 w323 w325 w327 w329 w331 w333 w335 w337 w339 w341 w343 w345 w347 w349 w351 w353 w355 w357 w359 w361 w363 w365 w367 w369 w371 w373 w375 w377 w379 w381 w383 w385 w387 w389 w391 w393 w395 w397 w399 w401 w403 w405 w407 w409 w411 w413 w415 w417 w419 w421 w423]
          tunnel: [w209 w212 w216 w221 w223 w225 w227 w229 w231 w233 w235 w237 w239 w241 w243 w245 w247 w249 w251 w253 w255 w257 w259 w261 w263 w265 w267 w269 w271 w273 w275 w277 w279 w281 w283 w285 w287 w289 w291 w293 w295 w297 w299 w301 w303 w305 w307 w309 w311 w313 w315 w317 w319 w321 w323 w325 w327 w329 w331 w333 w335 w337 w339 w341 w343 w345 w347 w349 w351 w353 w355 w357 w359 w361 w363 w365 w367 w369 w371 w373 w375 w377 w379 w381 w383 w385 w387 w389 w391 w393 w395 w397 w399 w401 w403 w405 w407 w409 w411 w413 w415 w417 w419 w421 w423] -> w117
          tunnel: w147 -> [w207 w211 w215 w219 _ _ _ _ _ _ _ _ _ _ _ _ _ _ _ _ _ _ _ _ _ _ _ _ _ _ _ _ _ _ _ _ _ _ _ _ _ _ _ _ _ _ _ _ _ _ _ _ _ _ _ _ _ _ _ _ _ _ _ _ _ _ _ _ _ _ _ _ _ _ _ _ _ _ _ _ _ _ _ _ _ _ _ _ _ _ _ _ _ _ _ _ _ _ _ _ _ _ _ _ _]
          frame "DOWN" {
            n116 = Add(x=w210, y=w207) -> (x+y=w209:sgl)
          }
          frame "LEFT" {
            n117 = Subtract(x=w214, y=w211) -> (x-y=w213:sgl)
          }
          frame "RIGHT" {
            n118 = Add(x=w218, y=w215) -> (x+y=w217:sgl)
          }
          frame "UP" {
            n119 = Subtract(x=w222, y=w219) -> (x-y=w221:sgl)
          }
          frame "ENTER (num pad)" {
          }
          frame "' (quote)" {
          }
          frame "END" {
          }
          frame "EQUALS" {
          }
          frame "ESCAPE" {
          }
          frame "GRAVE (`)" {
          }
          frame "HOME" {
          }
          frame "INSERT" {
          }
          frame "LBRACKET" {
          }
          frame "LCONTROL" {
          }
          frame "L ALT" {
          }
          frame "LSHIFT" {
          }
          frame "LWIN" {
          }
          frame "MINUS" {
          }
          frame "MULTIPLY" {
          }
          frame "NEXT" {
          }
          frame "NUMLOCK" {
          }
          frame "NUMPAD_0" {
          }
          frame "NUMPAD_1" {
          }
          frame "NUMPAD_2" {
          }
          frame "NUMPAD_3" {
          }
          frame "NUMPAD_4" {
          }
          frame "NUMPAD_5" {
          }
          frame "NUMPAD_6" {
          }
          frame "NUMPAD_7" {
          }
          frame "NUMPAD_8" {
          }
          frame "NUMPAD_9" {
          }
          frame "PAUSE" {
          }
          frame "PERIOD" {
          }
          frame "PRIOR (PG UP)" {
          }
          frame "RBRACKET" {
          }
          frame "RCONTROL" {
          }
          frame "RETURN" {
          }
          frame "R ALT" {
          }
          frame "RSHIFT" {
          }
          frame "RWIN" {
          }
          frame "SCROLL" {
          }
          frame "SEMICOLON" {
          }
          frame "SLASH" {
          }
          frame "SPACE" {
          }
          frame "SUBTRACT" {
          }
          frame "TAB" {
          }
          frame "DIVIDE" {
          }
          frame "DELETE" {
          }
          frame "DECIMAL" {
          }
          frame "COMMA" {
          }
          frame "CAPITAL" {
          }
          frame "BACKSLASH" {
          }
          frame "BACK" {
          }
          frame "ADD" {
          }
          frame "F15" {
          }
          frame "F14" {
          }
          frame "F13" {
          }
          frame "F12" {
          }
          frame "F11" {
          }
          frame "F10" {
          }
          frame "F9" {
          }
          frame "F8" {
          }
          frame "F7" {
          }
          frame "F6" {
          }
          frame "F5" {
          }
          frame "F4" {
          }
          frame "F3" {
          }
          frame "F2" {
          }
          frame "F1" {
          }
          frame "Z" {
          }
          frame "Y" {
          }
          frame "X" {
          }
          frame "W" {
          }
          frame "V" {
          }
          frame "U" {
          }
          frame "T" {
          }
          frame "S" {
          }
          frame "R" {
          }
          frame "Q" {
          }
          frame "P" {
          }
          frame "O" {
          }
          frame "N" {
          }
          frame "M" {
          }
          frame "L" {
          }
          frame "K" {
          }
          frame "J" {
          }
          frame "I" {
          }
          frame "H" {
          }
          frame "G" {
          }
          frame "F" {
          }
          frame "E" {
          }
          frame "D" {
          }
          frame "C" {
          }
          frame "B" {
          }
          frame "A" {
          }
          frame "9" {
          }
          frame "8" {
          }
          frame "7" {
          }
          frame "6" {
          }
          frame "5" {
          }
          frame "4" {
          }
          frame "3" {
          }
          frame "2" {
          }
          frame "1" {
          }
          frame "0" {
          }
        }
        n120 = property on="Previous File" class="Bool (strict)"(error in=w160, "Value"=w152) -> (error out=w159:errorcluster)  [unwired: 1 in, 1 out]
        n121 = Bundle(w136, w137, w122, w123, 0.0) -> (w124:cluster{dbl, dbl, dbl, dbl, dbl})  [unwired: 1 in]
        n122 = Divide(x=20, y=w148) -> (x/y=w146:sgl)
        n123 = Bundle("X"=w116, "Y"=w117) -> (w120:cluster{"X":sgl, "Y":sgl})  [unwired: 1 in]
        n124 = call "IMAQ Convert Rectangle to ROI (Polygon)"("Rectangle"=w124) -> ("ROI Descriptor"=w126:T14)  [unwired: 7 in, 2 out]
        n125 = property on="Save" class="Bool (strict)"(error in=w159, "Value"=w152) -> (error out=w158:errorcluster)  [unwired: 1 in, 1 out]
        n126 = property on="Export" class="Bool (strict)"("Value"=w152) -> ()  [unwired: 2 in, 2 out]
        n127 = property on="Image Out" class="ImageControl"("Image Center Position"=w120) -> ()  [unwired: 2 in, 2 out]
        n128 = property on="Image Preview" class="ImageControl"("ROI"=w126) -> ()  [unwired: 2 in, 2 out]
        n129 = property on="Save Next" class="Bool (strict)"(error in=w158, "Value"=w152) -> (error out=w157:errorcluster)  [unwired: 1 in, 1 out]
        n130 = property on="Discard" class="Bool (strict)"(error in=w157, "Value"=w152) -> (error out=w156:errorcluster)  [unwired: 1 in, 1 out]
        n131 = property on="Save Lines" class="Bool (strict)"(error in=w156, "Value"=w152) -> ()  [unwired: 1 in, 2 out]
        n132 = property on="Close" class="Bool (strict)"("Value"=w152) -> ()  [unwired: 2 in, 2 out]
        n133 = Bundle("Application Font", w146, w142, w142, w142, w142, w142, TRUE, w144) -> (w141:T15)  [unwired: 1 in]
        n134 = property on="Disable Flag" class="Bool (strict)"("Value"=w152) -> ()  [unwired: 2 in, 2 out]
        n135 = Bundle(w144, w141, w144, w144) -> (w98:T16)  [unwired: 1 in]
        n136 = Cluster To Array(cluster=w151) -> (array=w170:bool[])
        n137 = local read "Image Out"() -> (w97:T8)
        n138 = property on="Image Out" class="ImageControl"() -> ("ROI"=w100:T17)  [unwired: 2 in, 2 out]
        n139 = Unbundle By Name(w100) -> ("Contours"=w101:T18)
        n140 = call "IMAQ Clear Overlay"("Image"=w97) -> ("Image Out"=w114:T8)  [unwired: 9 in, 1 out]
        n141 = Initialize Array(0) -> (w103:i32[])  [unwired: 1 in]
        n142 = Array Size(array=w101) -> (size(s)=w102:i32)
        n143 = call "Next State.vi"("Buttons []"=w170, "States []"=w171) -> ("Enum"=w163:T2)
        n144 = event shown="[8] \"Sat-Log Slider\": Value Change" {
          selector: _ -> [_ _ _ _ _ _ _ _ _ _ _ _ _ _ _ _ _ _]
          dyn-events: _ -> [_ _ _ _ _ _ _ _ _ _ _ _ _ _ _ _ _ _]
          timeout: 5 -> [_ _ _ _ _ _ _ _ _ _ _ _ _ _ _ _ _ _]
          tunnel: w163 -> [w426 _ _ _ _ _ _ _ _ _ _ _ _ _ _ _ _ _]
          tunnel: [w426 MegaAwesome_States."Re-Calculated Values" MegaAwesome_States."Re-Calculated Values" MegaAwesome_States."Re-Calculated Values" MegaAwesome_States."Re-Calculated Values" MegaAwesome_States."Calculated Values" MegaAwesome_States."Re-Calculated Values" MegaAwesome_States."Re-Calculated Values" MegaAwesome_States."Re-Calculated Values" MegaAwesome_States."Re-Calculated Values" MegaAwesome_States."Read Data" MegaAwesome_States."Read Data" _ _ _ _ _ _] -> w162
          tunnel: w155 -> [w425 w427 w429 w431 w433 w435 w437 w462 w490 w514 _ w542 _ _ _ _ _ _]
          tunnel: [w425 w427 w429 w431 w433 w435 w437 w462 w490 w514 w533 w542 _ _ _ _ _ _] -> w154
          tunnel: w153 -> [_ _ _ _ _ _ _ _ _ _ w532 _ _ _ _ _ _ _]
          tunnel: w151 -> [_ _ _ _ _ _ _ _ _ _ _ _ _ _ _ _ _ _]
          event Timeout {
            n145 = event-data() -> ()  [unwired: 1 in, 2 out]
          }
          event "New: Dielectric": Value Change {
            n146 = event-data() -> ()  [unwired: 1 in, 5 out]
          }
          event "New: Length": Value Change {
            n147 = event-data() -> ()  [unwired: 1 in, 5 out]
          }
          event "New: Width": Value Change {
            n148 = event-data() -> ()  [unwired: 1 in, 5 out]
          }
          event "New: Temp": Value Change {
            n149 = event-data() -> ()  [unwired: 1 in, 5 out]
          }
          event "Num Pts Log", "Transport Style Controls", "Num Pts": Value Change {
            n150 = event-data() -> ()  [unwired: 1 in, 5 out]
          }
          event "Sat-Trans Slider": Value Change {
            n151 = event-data() -> ()  [unwired: 1 in, 5 out]
            n152 = local read "Sqrt-Sat"() -> (w461:cluster{dbl[], dbl[]}[])
            n153 = Decimate 1D Array(w461) -> (w445:cluster{dbl[], dbl[]}[], w446:cluster{dbl[], dbl[]}[])
            n154 = local read "Slider Min"() -> (w442:dbl)
            n155 = local read "Sat-Trans Slider"() -> (w440:dbl)
            n156 = Array To Cluster(array=w445) -> (cluster=w460:T19)
            n157 = local read "New: Dielectric"() -> (w455:dbl)
            n158 = local read "Num Pts"() -> (w438:dbl)
            n159 = local read "New: Width"() -> (w457:dbl)
            n160 = local read "New: Length"() -> (w456:dbl)
            n161 = Unbundle(w460) -> ("[0]"=w459:cluster{dbl[], dbl[]})  [unwired: 8 out]
            n162 = Absolute Value(x=w442) -> (abs(x)=w441:dbl)
            n163 = Unbundle(w459) -> (w443:dbl[], w458:dbl[])
            n164 = Add(x=w440, y=w441) -> (x+y=w439:dbl)
            n165 = Array Subset(array=w443, index=w439, length=w438) -> (w453:dbl[])
            n166 = local write "Sat Vg Array-Used"(w453) -> ()
            n167 = Array Subset(array=w458, index=w439, length=w438) -> (w454:dbl[])
            n168 = call "Mobility-Vt-Used Pts_Saturation.vi"("Width"=w457, "Length"=w456, "Dielectric (d)"=w455, "Sat Id Used"=w454, "Vg Used"=w453) -> ("Vt"=w449:dbl, "Mobility"=w450:dbl)  [unwired: 4 in, 1 out]
            n169 = local write "Index-Sat"(w439) -> ()
            n170 = local write "Sat Id-Used"(w454) -> ()
            n171 = Bundle(w453, w454) -> (w447:cluster{dbl[], dbl[]})  [unwired: 1 in]
            n172 = local read "Re-Calculated Values Cluster"() -> (w452:T9)
            n173 = Bundle By Name(cluster=w452, "Mobility-Sat"=w450, "Vt-Sat"=w449) -> (w451:T9)
            n174 = local write "Re-Calculated Values Cluster"(w451) -> ()
            n175 = Build Array (concatenate)(w445, w446, w447) -> (w444:cluster{dbl[], dbl[]}[])
            n176 = local write "Sqrt-Sat"(w444) -> ()
          }
          event "Lin-Trans Slider": Value Change {
            n177 = event-data() -> ()  [unwired: 1 in, 5 out]
            n178 = local read "Sqrt-Lin"() -> (w486:cluster{dbl[], dbl[]}[])
            n179 = Decimate 1D Array(w486) -> (w471:cluster{dbl[], dbl[]}[], w472:cluster{dbl[], dbl[]}[])
            n180 = local read "Slider Min"() -> (w468:dbl)
            n181 = Array To Cluster(array=w471) -> (cluster=w485:T19)
            n182 = local read "Lin-Trans Slider"() -> (w466:dbl)
            n183 = local read "New: Dielectric"() -> (w479:dbl)
            n184 = local read "Num Pts"() -> (w482:dbl)
            n185 = local read "New: Width"() -> (w481:dbl)
            n186 = local read "New: Length"() -> (w480:dbl)
            n187 = local read "Lin Vd"() -> (w463:dbl)
            n188 = Unbundle(w485) -> ("[0]"=w484:cluster{dbl[], dbl[]})  [unwired: 8 out]
            n189 = Absolute Value(x=w468) -> (abs(x)=w467:dbl)
            n190 = Unbundle(w484) -> (w469:dbl[], w483:dbl[])
            n191 = Add(x=w466, y=w467) -> (x+y=w465:dbl)
            n192 = Array Subset(array=w469, index=w465, length=w482) -> (w477:dbl[])
            n193 = local write "Lin-Vg Array-Used"(w477) -> ()
            n194 = Array Subset(array=w483, index=w465, length=w482) -> (w478:dbl[])
            n195 = call "Mobility-Vt-Used Pts_Linear.vi"("Width"=w481, "Length"=w480, "Vd"=w463, "Dielectric (d)"=w479, "Id Used"=w478, "Vg Used"=w477) -> ("Mobility"=w474:dbl)  [unwired: 3 in, 2 out]
            n196 = local write "Index-Lin"(w465) -> ()
            n197 = local write "Lin Id-Used"(w478) -> ()
            n198 = Bundle(w477, w478) -> (w473:cluster{dbl[], dbl[]})  [unwired: 1 in]
            n199 = local read "Re-Calculated Values Cluster"() -> (w476:T9)
            n200 = Bundle By Name(cluster=w476, "Moblitity-Lin"=w474) -> (w475:T9)
            n201 = local write "Re-Calculated Values Cluster"(w475) -> ()
            n202 = Build Array (concatenate)(w471, w472, w473) -> (w470:cluster{dbl[], dbl[]}[])
            n203 = local write "Sqrt-Lin"(w470) -> ()
          }
          event "Sat-Log Slider": Value Change {
            n204 = event-data() -> ()  [unwired: 1 in, 5 out]
            n205 = local read "Sat-Log"() -> (w493:cluster{dbl[], dbl[]}[])
            n206 = Decimate 1D Array(w493) -> (w500:cluster{dbl[], dbl[]}[], w501:cluster{dbl[], dbl[]}[])
            n207 = local read "Slider Min"() -> (w497:dbl)
            n208 = Array To Cluster(array=w500) -> (cluster=w510:T19)
            n209 = property on="Sat-Log" class="XYGraph (strict)"("Active Plot"=2, "Plot.Fill/Pt. Color"=u32 6618880, "Plot.Point Style"=11) -> ()  [unwired: 2 in, 2 out]
            n210 = local read "Num Pts Log"() -> (w507:dbl)
            n211 = local read "Sat-Log Slider"() -> (w495:dbl)
            n212 = Unbundle(w510) -> ("[0]"=w509:cluster{dbl[], dbl[]})  [unwired: 8 out]
            n213 = Absolute Value(x=w497) -> (abs(x)=w496:dbl)
            n214 = Unbundle(w509) -> (w498:dbl[], w508:dbl[])
            n215 = Add(x=w495, y=w496) -> (x+y=w492:dbl)
            n216 = Array Subset(array=w498, index=w492, length=w507) -> (w505:dbl[])
            n217 = Array Subset(array=w508, index=w492, length=w507) -> (w506:dbl[])
            n218 = local write "Vg Array-Log-Used"(w505) -> ()
            n219 = local write "IndexLog-Sat"(w492) -> ()
            n220 = Bundle(w505, w506) -> (w491:cluster{dbl[], dbl[]})  [unwired: 1 in]
            n221 = call "STS-Used.vi"("Id Used"=w506, "Vg-Used"=w505) -> ("STS"=w502:dbl)  [unwired: 9 in]
            n222 = local write "Sat Id-Log-Used"(w506) -> ()
            n223 = local read "Re-Calculated Values Cluster"() -> (w504:T9)
            n224 = Bundle By Name(cluster=w504, "STS"=w502) -> (w503:T9)
            n225 = local write "Re-Calculated Values Cluster"(w503) -> ()
            n226 = Build Array (concatenate)(w500, w501, w491) -> (w499:cluster{dbl[], dbl[]}[])
            n227 = local write "Sat-Log"(w499) -> ()
          }
          event "Lin-Log Slider": Value Change {
            n228 = event-data() -> ()  [unwired: 1 in, 5 out]
            n229 = local read "Lin-Log"() -> (w518:cluster{dbl[], dbl[]}[])
            n230 = Decimate 1D Array(w518) -> (w524:cluster{dbl[], dbl[]}[], w525:cluster{dbl[], dbl[]}[])
            n231 = local read "Slider Min"() -> (w521:dbl)
            n232 = Array To Cluster(array=w524) -> (cluster=w531:T19)
            n233 = local read "Num Pts Log"() -> (w528:dbl)
            n234 = property on="Lin-Log" class="XYGraph (strict)"("Active Plot"=2, "Plot.Fill/Pt. Color"=u32 6618880, "Plot.Point Style"=11) -> ()  [unwired: 2 in, 2 out]
            n235 = local read "Lin-Log Slider"() -> (w519:dbl)
            n236 = Unbundle(w531) -> ("[0]"=w530:cluster{dbl[], dbl[]})  [unwired: 8 out]
            n237 = Absolute Value(x=w521) -> (abs(x)=w520:dbl)
            n238 = Unbundle(w530) -> (w522:dbl[], w529:dbl[])
            n239 = Add(x=w519, y=w520) -> (x+y=w517:dbl)
            n240 = Array Subset(array=w522, index=w517, length=w528) -> (w526:dbl[])
            n241 = local write "Lin-Vg Array-Log Used"(w526) -> ()
            n242 = Array Subset(array=w529, index=w517, length=w528) -> (w527:dbl[])
            n243 = local write "IndexLog-Sat"(w517) -> ()
            n244 = Bundle(w526, w527) -> (w516:cluster{dbl[], dbl[]})  [unwired: 1 in]
            n245 = local write "Lin Id-Log Used"(w527) -> ()
            n246 = Build Array (concatenate)(w524, w525, w516) -> (w523:cluster{dbl[], dbl[]}[])
            n247 = local write "Lin-Log"(w523) -> ()
          }
          event "Index Array": Value Change {
            n248 = event-data() -> ()  [unwired: 1 in, 5 out]
            n249 = Strip Path(path=w532) -> (stripped path=w538:path)  [unwired: 1 out]
            n250 = local write "Transfer Folder"(w538) -> ()
            n251 = List Folder(path=w538) -> (filenames=w534:string[])  [unwired: 3 in, 3 out]
            n252 = local read "Index Array"() -> (w533:u16)
            n253 = Path To String(path=w538) -> (string=w539:string)
            n254 = Index Array(array=w534, index=w533) -> (element=w540:string)
            n255 = Concatenate Strings(w539, "\\", w540) -> (w536:string)
            n256 = String To Path(string=w536) -> (path=w535:path)
            n257 = local write "Transfer File"(w535) -> ()
          }
          event "Transfer File": Value Change {
            n258 = event-data() -> ()  [unwired: 1 in, 5 out]
          }
          event "Remove Button": Mouse Down {
            w544 = 0
            n259 = event-data() -> ()  [unwired: 1 in, 5 out]
            n260 = property on="Image Out" class="ImageControl"() -> ("ROI"=w554:T17)  [unwired: 2 in, 2 out]
            n261 = Unbundle(w554) -> ("Global Rectangle"=w545:i32[], "Contours"=w547:T18)
            n262 = Reverse 1D Array(array=w545) -> (reversed array=w546:i32[])
            n263 = Reverse 1D Array(array=w547) -> (reversed array=w548:T18)
            n264 = Delete From Array(array=w546, index=w544) -> (array with subset deleted=w549:i32[])  [unwired: 1 in, 1 out]
            n265 = Delete From Array(array=w548, index=w544) -> (array with subset deleted=w550:T18)  [unwired: 1 in, 1 out]
            n266 = Reverse 1D Array(array=w549) -> (reversed array=w551:i32[])
            n267 = Reverse 1D Array(array=w550) -> (reversed array=w552:T18)
            n268 = Bundle(w551, w552) -> (w553:T20)  [unwired: 1 in]
            n269 = property on="Image Out" class="ImageControl"("ROI"=w553) -> ()  [unwired: 2 in, 2 out]
          }
          event "Undo Button": Mouse Down {
            n270 = event-data() -> ()  [unwired: 1 in, 5 out]
            n271 = invoke on="Image Out" class="ImageControl" method="Clear ROI"() -> ()  [unwired: 3 in, 3 out]
          }
          event "Image Folder": Value Change {
            n272 = event-data() -> ()  [unwired: 1 in, 5 out]
            n273 = local read "Image File"() -> (w555:path)
            n274 = call "Vision Acquisition"("Image Path"=w555) -> ("Image Out"=w556:T8)  [unwired: 25 in, 1 out]
            n275 = local write "Image Preview"(w556) -> ()
            n276 = local write "Image Out"(w556) -> ()
          }
          event "Zoom": Value Change {
            n277 = event-data() -> ()  [unwired: 1 in, 5 out]
            n278 = local read "Zoom"() -> (w558:i32)
            n279 = Bundle("Zoom"=w558, "Zoom"=w558) -> (w557:cluster{"Zoom":i32, "Zoom":i32})  [unwired: 1 in]
            n280 = property on="Image Out" class="ImageControl"("ZoomInteger"=w557) -> ()  [unwired: 2 in, 2 out]
          }
          event "Image Out": Mouse Enter {
            n281 = event-data() -> ()  [unwired: 1 in, 3 out]
            n282 = call "Simulate_Keyboard.vi"("Action"=0, "Virtual Key"=162) -> ()  [unwired: 7 in, 1 out]
          }
          event "Image Out": Mouse Leave {
            n283 = event-data() -> ()  [unwired: 1 in, 3 out]
            n284 = flat-sequence {
              frame #0 {
                n285 = Wait (ms)(milliseconds to wait=10) -> ()  [unwired: 1 out]
              }
              frame #1 {
                n286 = call "Simulate_Keyboard.vi"("Action"=2, "Virtual Key"=162) -> ()  [unwired: 7 in, 1 out]
              }
            }
          }
        }
        n287 = Build Array(0.505025, 0.252522, 0.127742, 0.050345, 0.031129) -> (w110:dbl[])
        n288 = Array Subset(array=w110, index="Magnification", length=1) -> (w112:dbl[])
        n289 = To Double Precision Float(number=w112) -> (double precision float=w113:dbl[])
        n290 = for {
          N: w102 -> [_]
          shift-right: [w197] -> _
          shift-left: w101 -> [w197]
          shift-right: [w173] -> w88
          shift-left: w103 -> [w195]
          tunnel: w113 -> [w194]
          shift-right: [w191] -> _
          shift-left: w114 -> [w193]
          tunnel: w98 -> [w187]
          i -> [w190]
          n291 = Index Array(array=w197, index=w190) -> (element=w206:T21)
          n292 = Unbundle(w206) -> ("Points"=w205:i32[])  [unwired: 2 out]
          n293 = Array To Cluster(array=w205) -> (cluster=w204:T22)
          n294 = Unbundle(w204) -> ("Points[0]"=w186:i32, "Points[1]"=w183:i32, "Points[2]"=w196:i32, "Points[3]"=w202:i32)  [unwired: 5 out]
          n295 = Add(x=w186, y=10) -> (x+y=w184:i32)
          n296 = Subtract(x=w183, y=w202) -> (x-y=w201:i32)
          n297 = Subtract(x=w186, y=w196) -> (x-y=w203:i32)
          n298 = Square(x=w201) -> (x^2=w199:i32)
          n299 = Square(x=w203) -> (x^2=w200:i32)
          n300 = Add(x=w200, y=w199) -> (x+y=w198:i32)
          n301 = Square Root(x=w198) -> (sqrt(x)=w177:dbl)
          n302 = Multiply(x=w177, y=0.5) -> (x*y=w180:dbl)
          n303 = Add(x=w180, y=w183) -> (x+y=w182:dbl)
          n304 = Bundle(w184, w182) -> (w192:cluster{i32, dbl})  [unwired: 1 in]
          n305 = Multiply(x=w177, y=w194) -> (x*y=w176:dbl[])
          n306 = Index Array(array=w176) -> (element=w189:dbl)  [unwired: 1 in]
          n307 = Number To Fractional String(number=w189, precision (6)=0) -> (F-format string=w188:string)  [unwired: 2 in]
          n308 = call "IMAQ Overlay Text"("BG Color (Transparent)"=u32 0, "Text Color (black)"=u32 16448250, "Font, Size & Style"=w187, "String"=w188, "Origin"=w192, "Image"=w193) -> ("Image Out"=w191:T8)  [unwired: 4 in, 1 out]
          n309 = Build Array (concatenate)(w195, w176) -> (w174:dbl[])
          n310 = To Long Integer(number=w174) -> (32bit integer=w173:i32[])
        }
        "Distances" <- w88
        n311 = Add Array Elements(numeric array=w88) -> (sum=w99:i32)
        n312 = local write "Total Width"(w99) -> ()
      }
      frame "Read Data" {
        n313 = call "IMAQ Dispose"("All Images? (No)"=TRUE) -> ()  [unwired: 5 in, 1 out]
        n314 = case shown="True" "Disable Flag" {
          tunnel: w609 -> [_ w634]
          tunnel: [w630 w631] -> w608
          tunnel: w606 -> [w630 _]
          frame False {
          }
          frame True {
            n315 = local read "Transfer Folder"() -> (w633:path)
            n316 = List Folder(path=w633) -> (filenames=w635:string[])  [unwired: 3 in, 3 out]
            n317 = Index Array(array=w635, index=w634) -> (element=w632:string)
            n318 = Build Path(base path=w633, name or relative path=w632) -> (appended path=w631:path)
            n319 = local write "Transfer File"(w631) -> ()
          }
        }
        n320 = call "Recorded Values.vi"("Path"=w608) -> ("Recorded Char"=→"Recorded Values Cluster":T9, "Recorded Prop"=w621:T1, "Fabrication Prop"=w619:T4)  [unwired: 8 in]
        n321 = Strip Path(path=w608) -> (stripped path=w618:path, name=w617:string)
        n322 = local write "Fabrication Prop"(w619) -> ()
        n323 = local write "Recorded Prop"(w621) -> ()
        n324 = Unbundle By Name(w621) -> ("Date Recorded"=→"Date Recorded":string, "Index"=w620:string, "Length"=w614:dbl, "Width"=w613:dbl)  [unwired: 1 out]
        n325 = Unbundle By Name(w621) -> ("Sample Temp"=w623:dbl)
        n326 = Unbundle By Name(w619) -> ("Dielectric (nm)"=w615:dbl, "Comments"=w616:string, "Date Created"=→"Date Created":string)
        n327 = List Folder(path=w618) -> (filenames=w612:string[])  [unwired: 3 in, 3 out]
        n328 = local write "Rec: Dielectric (d)"(w615) -> ()
        n329 = local write "Index"(w620) -> ()
        n330 = local write "Rec: Length"(w614) -> ()
        n331 = local write "Rec: Width"(w613) -> ()
        n332 = Equal To 0?(x=w623) -> (x = 0?=w626:bool)
        n333 = Number To Decimal String(number=w623) -> (decimal integer string=w627:string)  [unwired: 1 in]
        n334 = local write "Comments:"(w616) -> ()
        n335 = Search 1D Array(1D array=w612, element=w617) -> (index of element=w611:i32)  [unwired: 1 in]
        n336 = Equal?(x="", y=w627) -> (x = y?=w625:bool)
        n337 = Index Array(array=w612, index=w611) -> (element=→"Data Name:":string)
        n338 = local write "New: Width"(w613) -> ()
        n339 = local write "New: Length"(w614) -> ()
        n340 = local write "Index Array"(w611) -> ()
        n341 = Or(x=w626, y=w625) -> (x .or. y?=w624:bool)
        n342 = local write "New: Dielectric"(w615) -> ()
        n343 = case shown="True" w624 {
          tunnel: [w636 w637] -> w605
          tunnel: w623 -> [w636 _]
          frame False {
          }
          frame True {
            n344 = local read "Room Temp"() -> (w637:dbl)
          }
        }
        n345 = local write "New: Temp"(w605) -> ()
        n346 = Bundle By Name(cluster=w621, "Sample Temp"=w605) -> (w622:T1)
        n347 = local write "Rec: Temp"(w605) -> ()
        n348 = local write "Recorded Prop"(w622) -> ()
      }
      frame "Calculated Values" {
        n349 = local read "Image Center X"() -> (w639:i32)
        n350 = call "Image from TRF Display.vi"("Image Center X"=w639, "No Image File"=w684, "Image Folder"=w685, "Transfer File"=w654) -> ("Image Preview"=w646:T8, "Image Out"=w647:T8, "Image File"=w648:path, "Image Name"=→"Image Name":string, "ROI File"=w643:path)  [unwired: 3 in]
        n351 = invoke on="Image Out" class="ImageControl" method="Clear ROI"() -> ()  [unwired: 3 in, 3 out]
        n352 = local write "Image File"(w648) -> ()
        n353 = local write "Image Out"(w647) -> ()
        n354 = local write "Image Preview"(w646) -> ()
        n355 = call <vilib>:"Check if File or Folder Exists.vi"("path"=w643) -> ("file or folder exists?"=w644:bool, "dup path"=w645:path)  [unwired: 8 in, 1 out]
        n356 = case shown="True" w644 {
          tunnel: w645 -> [_ w705]
          frame False {
          }
          frame True {
            n357 = Read from Text File(file (use dialog)=w705) -> (text=w709:string)  [unwired: 3 in, 3 out]
            n358 = property on="Image Out" class="ImageControl"() -> ("ROI"=w706:T17)  [unwired: 2 in, 2 out]
            n359 = Unflatten From String(type=w706, binary string=w709) -> (value=w707:T17, error out=w708:errorcluster)  [unwired: 3 in, 1 out]
            n360 = property on="Image Out" class="ImageControl"(error in=w708, "ROI"=w707) -> ()  [unwired: 1 in, 2 out]
          }
        }
        n361 = call "TRF to TSP Plot_09_21_12a_JW.vi"("Transport Graph Properties"="Transport Style Controls", "No Transport File"=w649, "Transport Folder"=w650, "Transfer File"=w654) -> ("Transport"=w655:cluster{ext[], ext[]}[], "Transport File"=→"Transport\nFile":path, "Transport Name"=→"Transport Name:":string)  [unwired: 5 in]
        "Transport" <- w655
        n362 = Array Size(array=w655) -> (size(s)=w653:i32)
        n363 = local read "Image Center X"() -> (w640:i32)
        n364 = for {
          N: w653 -> [_]
          tunnel: "Transport Style Controls" -> [w713]
          i -> [w712]
          n365 = Unbundle By Name(w713) -> ("Transport Line Size"=w710:u16, "Transport Line Color"=w711:u32)
          n366 = property on="Transport" class="XYGraph (strict)"("Active Plot"=w712, "Plot.Plot Color"=w711, "Plot.Line Width"=w710) -> ()  [unwired: 2 in, 2 out]
        }
        n367 = local read "Recorded Prop"() -> (w687:T1)
        n368 = local read "Fabrication Prop"() -> (w694:T4)
        n369 = Bundle("Image Center X"=w640, 0) -> (w642:cluster{"Image Center X":i32, i32})  [unwired: 1 in]
        n370 = property on="Image Out" class="ImageControl"("Image Center Position"=w642) -> ()  [unwired: 2 in, 2 out]
        n371 = local read "Calculated Values Cluster"() -> (w704:T9)
        n372 = call "Mobility-Vt Calculator-File.vi"("NumPts"=w689, "Path"=w654) -> ("Used Points"=w682:T23, "Graph Cluster"=w672:T24, "Lin Vd"=w657:dbl, "Output"=w702:T25)  [unwired: 6 in]
        n373 = call "STS Calculator-File.vi"("NumPts"=w688, "Path"=w654) -> ("Used Points"=w677:T26, "XY Graph-Sat"=w661:cluster{dbl[], dbl[]}[], "XY Graph-Lin"=w658:cluster{dbl[], dbl[]}[], "Ouput"=w697:cluster{"STS-Sat":dbl, "STS-Lin":dbl})  [unwired: 6 in]
        n374 = Unbundle By Name(w694) -> ("Dielectric (nm)"=w692:dbl)
        n375 = Unbundle By Name(w687) -> ("Sample Temp"=w686:dbl)
        n376 = Unbundle By Name(w702) -> ("Mobility-Sat"=w701:dbl, "Vt-Sat"=w693:dbl, "Mobility-Lin"=w700:dbl, "Off I-Sat"=w699:dbl, "On/Off I-Sat"=w698:dbl)  [unwired: 1 out]
        n377 = local write "Lin Vd"(w657) -> ()
        n378 = Unbundle By Name(w697) -> ("STS-Sat"=w691:dbl)  [unwired: 1 out]
        n379 = local write "Sat-Log"(w661) -> ()
        n380 = local write "Lin-Log"(w658) -> ()
        n381 = call "Trap Density_VT.vi"("VT"=w693, "Dielectric"=w692) -> ("Trap Density-VT"=w696:dbl)
        n382 = call "Trap Density_STS.vi"("Temp (T) [K]"=w686, "S.T.S. (S)"=w691, "Dielectric"=w692) -> ("Trap Density (N)"=w695:dbl)  [unwired: 8 in]
        n383 = Bundle By Name(cluster=w704, "Mobility-Sat"=w701, "Moblitity-Lin"=w700, "On/Off"=w698, "Off Current"=w699, "Vt-Sat"=w693, "STS"=w691, "Trap Density-VT"=w696, "Trap Density-STS"=w695) -> (w703:T9)
        n384 = Unbundle By Name(w677) -> ("Sat Vg Used"=w676:dbl[], "Sat Log(Id) Used"=w675:dbl[], "Lin Vg Used"=w674:dbl[], "Lin Log(Id) Used"=w673:dbl[], "STS Index-Sat"=w659:dbl, "STS Index-Lin"=w660:dbl)
        n385 = Unbundle By Name(w682) -> ("Sat Vg Used"=w681:dbl[], "Sat Sqrt(Id) Used"=w680:dbl[], "Lin Vg Used"=w679:dbl[], "Lin Sqrt(Id) Used"=w678:dbl[], "Index-Lin"=w668:dbl, "Index-Sat"=w667:dbl)
        n386 = local write "Vg Array-Log-Used"(w676) -> ()
        n387 = local write "Sat Id-Log-Used"(w675) -> ()
        n388 = local write "Lin-Vg Array-Log Used"(w674) -> ()
        n389 = local write "Lin Id-Log Used"(w673) -> ()
        n390 = local write "IndexLog-Sat"(w659) -> ()
        n391 = local write "Index-Lin"(w660) -> ()
        n392 = local write "Calculated Values Cluster"(w703) -> ()
        n393 = local write "Sat Vg Array-Used"(w681) -> ()
        n394 = local write "Sat Id-Used"(w680) -> ()
        n395 = local write "Lin-Vg Array-Used"(w679) -> ()
        n396 = local write "Lin Id-Used"(w678) -> ()
        n397 = local write "Index-Sat"(w667) -> ()
        n398 = local write "Index-Lin"(w668) -> ()
        n399 = local write "Lin-Log Slider"(w660) -> ()
        n400 = local write "Sat-Log Slider"(w659) -> ()
        n401 = local write "Sat-Trans Slider"(w667) -> ()
        n402 = local write "Lin-Trans Slider"(w668) -> ()
        n403 = Unbundle By Name(w672) -> ("Raw Sat"=w666:cluster{dbl[], dbl[]}[], "Sqrt Sat"=w669:cluster{dbl[], dbl[]}[], "Raw Lin"=w671:cluster{dbl[], dbl[]}[], "Sqrt Lin"=w670:cluster{dbl[], dbl[]}[])
        n404 = Index Array(array=w666) -> (element=w665:cluster{dbl[], dbl[]})  [unwired: 1 in]
        n405 = Unbundle(w665) -> (w664:dbl[])  [unwired: 1 out]
        n406 = Array Max & Min(array=w664) -> (max value=w663:dbl, min value=w662:dbl)  [unwired: 2 out]
        n407 = property on="Sat-Trans Slider" class="Slide (strict)"("Scale.Maximum"=w663, "Scale.Minimum"=w662) -> ()  [unwired: 2 in, 2 out]
        n408 = property on="Lin-Trans Slider" class="Slide (strict)"("Scale.Maximum"=w663, "Scale.Minimum"=w662) -> ()  [unwired: 2 in, 2 out]
        n409 = property on="Sat-Log Slider" class="Slide (strict)"("Scale.Maximum"=w663, "Scale.Minimum"=w662) -> ()  [unwired: 2 in, 2 out]
        n410 = property on="Lin-Log Slider" class="Slide (strict)"("Scale.Maximum"=w663, "Scale.Minimum"=w662) -> ()  [unwired: 2 in, 2 out]
        n411 = local write "Slider Max"(w663) -> ()
        n412 = local write "Slider Min"(w662) -> ()
        n413 = local write "Raw- Sat"(w666) -> ()
        n414 = local write "Raw- Lin"(w671) -> ()
        n415 = local write "Sqrt-Sat"(w669) -> ()
        n416 = local write "Sqrt-Lin"(w670) -> ()
      }
      frame "Re-Calculated Values" {
        n417 = local read "Vg Array-Log-Used"() -> (w722:dbl[])
        n418 = local read "Sat Vg Array-Used"() -> (w730:dbl[])
        n419 = local read "Lin-Vg Array-Used"() -> (w736:dbl[])
        n420 = local read "Sat Id-Log-Used"() -> (w721:dbl[])
        n421 = local read "New: Dielectric"() -> (w734:dbl)
        n422 = local read "New: Dielectric"() -> (w719:dbl)
        n423 = local read "New: Length"() -> (w733:dbl)
        n424 = local read "New: Length"() -> (w729:dbl)
        n425 = local read "New: Width"() -> (w732:dbl)
        n426 = local read "New: Width"() -> (w728:dbl)
        n427 = local read "Lin Id-Used"() -> (w735:dbl[])
        n428 = local read "Sat Id-Used"() -> (w727:dbl[])
        n429 = local read "Re-Calculated Values Cluster"() -> (w738:T9)
        n430 = local read "New: Dielectric"() -> (w718:dbl)
        n431 = local read "New: Temp"() -> (w717:dbl)
        n432 = local read "Lin Vd"() -> (w714:dbl)
        n433 = call "Mobility-Vt-Used Pts_Saturation.vi"("Width"=w728, "Length"=w729, "Dielectric (d)"=w719, "Sat Id Used"=w727, "Vg Used"=w730) -> ("Vt"=w725:dbl, "Mobility"=w726:dbl)  [unwired: 4 in, 1 out]
        n434 = call "STS-Used.vi"("Id Used"=w721, "Vg-Used"=w722) -> ("STS"=w720:dbl)  [unwired: 9 in]
        n435 = call "Mobility-Vt-Used Pts_Linear.vi"("Width"=w732, "Length"=w733, "Vd"=w714, "Dielectric (d)"=w734, "Id Used"=w735, "Vg Used"=w736) -> ("Mobility"=w731:dbl)  [unwired: 3 in, 2 out]
        n436 = call "Trap Density_VT.vi"("VT"=w725, "Dielectric"=w719) -> ("Trap Density-VT"=w724:dbl)
        n437 = call "Trap Density_STS.vi"("Temp (T) [K]"=w717, "S.T.S. (S)"=w720, "Dielectric"=w718) -> ("Trap Density (N)"=w716:dbl)  [unwired: 8 in]
        n438 = Bundle By Name(cluster=w738, "Mobility-Sat"=w726, "Moblitity-Lin"=w731, "Vt-Sat"=w725, "STS"=w720, "Trap Density-VT"=w724, "Trap Density-STS"=w716) -> (w737:T9)
        n439 = local write "Re-Calculated Values Cluster"(w737) -> ()
      }
      frame "Next File" {
        n440 = call "IMAQ Dispose"("All Images? (No)"=TRUE) -> ()  [unwired: 5 in, 1 out]
        n441 = Strip Path(path=w755) -> (stripped path=w746:path, name=w753:string)
        n442 = local write "Transfer Folder"(w746) -> ()
        n443 = List Folder(path=w746) -> (filenames=w740:string[])  [unwired: 3 in, 3 out]
        n444 = Array Size(array=w740) -> (size(s)=w752:i32)
        n445 = Search 1D Array(1D array=w740, element=w753) -> (index of element=w750:i32)  [unwired: 1 in]
        n446 = Decrement(x=w752) -> (x-1=w751:i32)
        n447 = Equal?(x=w751, y=w750) -> (x = y?=w749:bool)
        n448 = case shown="True" w749 {
          tunnel: w742 -> [w757 _]
          tunnel: [w756 0] -> w741
          frame False {
            n449 = Increment(x=w757) -> (x+1=w756:i32)
          }
          frame True {
          }
        }
        n450 = Path To String(path=w746) -> (string=w747:string)
        n451 = Index Array(array=w740, index=w741) -> (element=w748:string)
        n452 = Concatenate Strings(w747, "\\", w748) -> (w744:string)
        n453 = String To Path(string=w744) -> (path=w743:path)
        n454 = local write "Transfer File"(w743) -> ()
      }
      frame "Previous File" {
        n455 = call "IMAQ Dispose"("All Images? (No)"=TRUE) -> ()  [unwired: 5 in, 1 out]
        n456 = Strip Path(path=w766) -> (stripped path=w763:path, name=w774:string)
        n457 = local write "Transfer Folder"(w763) -> ()
        n458 = List Folder(path=w763) -> (filenames=w767:string[])  [unwired: 3 in, 3 out]
        n459 = Array Size(array=w767) -> (size(s)=w761:i32)
        n460 = Search 1D Array(1D array=w767, element=w774) -> (index of element=w773:i32)  [unwired: 1 in]
        n461 = Decrement(x=w761) -> (x-1=w760:i32)
        n462 = Equal To 0?(x=w773) -> (x = 0?=w772:bool)
        n463 = case shown="True" w772 {
          tunnel: w765 -> [w777 _]
          tunnel: [w776 w778] -> w764
          tunnel: w760 -> [_ w778]
          frame False {
            n464 = Decrement(x=w777) -> (x-1=w776:i32)
          }
          frame True {
          }
        }
        n465 = Path To String(path=w763) -> (string=w762:string)
        n466 = Index Array(array=w767, index=w764) -> (element=w771:string)
        n467 = Concatenate Strings(w762, "\\", w771) -> (w769:string)
        n468 = String To Path(string=w769) -> (path=w768:path)
        n469 = local write "Transfer File"(w768) -> ()
      }
      frame "Discard File" {
        n470 = flat-sequence {
          tunnel: w784 -> [w787]
          tunnel: [w787] -> w783
          tunnel: [w786] -> w780
          tunnel: w783 -> [w799]
          tunnel: w780 -> [w792]
          tunnel: [w791] -> w779
          frame #0 {
            n471 = Strip Path(path=w787) -> (stripped path=w790:path, name=w789:string)
            n472 = List Folder(path=w790) -> (filenames=w788:string[])  [unwired: 3 in, 3 out]
            n473 = Search 1D Array(1D array=w788, element=w789) -> (index of element=w786:i32)  [unwired: 1 in]
          }
          frame #1 {
            n474 = Strip Path(path=w799) -> (stripped path=w800:path, name=w798:string)
            n475 = String Subset(string=w798, offset (0)=0, length (rest)=1) -> (substring=w795:string)
            n476 = Equal?(x=w795, y="X") -> (x = y?=w793:bool)
            n477 = case shown="True" w793 {
              tunnel: w800 -> [w807 _]
              tunnel: w799 -> [w803 _]
              tunnel: w798 -> [w802 _]
              tunnel: w792 -> [w801 w811]
              tunnel: [w801 w810] -> w791
              frame False {
                n478 = Path To String(path=w807) -> (string=w806:string)
                n479 = Concatenate Strings(w806, "\\", "X_", w802) -> (w805:string)
                n480 = String To Path(string=w805) -> (path=w804:path)
                n481 = Move(source path=w803, 10:w804) -> ()  [unwired: 3 in, 3 out]
              }
              frame True {
                n482 = Increment(x=w811) -> (x+1=w810:i32)
              }
            }
          }
        }
        n483 = property on="Disable Flag" class="Bool (strict)"("Value"=TRUE) -> ()  [unwired: 2 in, 2 out]
        n484 = call "IMAQ Dispose"("All Images? (No)"=TRUE) -> ()  [unwired: 5 in, 1 out]
      }
      frame "Save" {
        n485 = stacked-sequence {
          seq-local: [w827 _] -> [_ w1324]
          seq-local: [w826 _] -> [_ w1322]
          tunnel: w819 -> [w828 w1325]
          frame #0 {
            # "Saves each Re-calculated parameter in sequence"
            n486 = stacked-sequence {
              tunnel: [_ _ _ _ _ _ _ _ _ _ _ _ _ w1292] -> w826
              tunnel: w828 -> [w848 _ _ _ _ _ _ _ _ _ _ _ _ _]
              frame #0 {
                n487 = call-poly <vilib>:"Read From Spreadsheet File.vi"("file path (dialog if empty)"=w848) -> ("all rows"=w847:string[][])  [unwired: 6 in, 4 out]
                n488 = Array Size(array=w847) -> (size(s)=w852:i32[])
                n489 = Array Subset(array=w847, index (row)=0, index (col)=0, length (col)=3) -> (w856:string[][])  [unwired: 1 in]
                n490 = Index Array(array=w852, index=0) -> (element=w850:i32)
                n491 = Reshape Array(w856, w850) -> (w849:string[])
                n492 = Search 1D Array(1D array=w849, element="Dielectric (nm):") -> (index of element=w859:i32)  [unwired: 1 in]
                n493 = Equal?(x=w859, y=-1) -> (x = y?=w858:bool)
                n494 = case shown="False" w858 {
                  tunnel: w847 -> [w867 w871]
                  tunnel: w859 -> [w863 _]
                  tunnel: [w862 w871] -> w857
                  frame False {
                    n495 = local read "Rec: Dielectric (d)"() -> (w869:dbl)
                    n496 = Number To Fractional String(number=w869) -> (F-format string=w864:string)  [unwired: 3 in]
                    n497 = Divide(x=w863, y=3) -> (x/y=w866:dbl)
                    n498 = To Word Integer(number=w866) -> (16bit integer=w865:i16)
                    n499 = Replace Array Subset(array=w867, new element=w864, index (row)=w865, index (col)=1) -> (w862:string[][])
                  }
                  frame True {
                  }
                }
                n500 = local write "Save Array"(w857) -> ()
              }
              frame #1 {
                n501 = local read "Save Array"() -> (w873:string[][])
                n502 = Array Size(array=w873) -> (size(s)=w876:i32[])
                n503 = Array Subset(array=w873, index (row)=0, index (col)=0, length (col)=3) -> (w880:string[][])  [unwired: 1 in]
                n504 = Index Array(array=w876, index=0) -> (element=w874:i32)
                n505 = Reshape Array(w880, w874) -> (w872:string[])
                n506 = Search 1D Array(1D array=w872, element="Comments:") -> (index of element=w883:i32)  [unwired: 1 in]
                n507 = Equal?(x=w883, y=-1) -> (x = y?=w882:bool)
                n508 = case shown="False" w882 {
                  tunnel: w873 -> [w891 w894]
                  tunnel: w883 -> [w888 _]
                  tunnel: [w887 w894] -> w881
                  frame False {
                    n509 = local read "New: Comments"() -> (w886:string)
                    n510 = Divide(x=w888, y=3) -> (x/y=w890:dbl)
                    n511 = To Word Integer(number=w890) -> (16bit integer=w889:i16)
                    n512 = Replace Array Subset(array=w891, new element=w886, index (row)=w889, index (col)=1) -> (w887:string[][])
                  }
                  frame True {
                  }
                }
                n513 = local write "Save Array"(w881) -> ()
              }
              frame #2 {
                n514 = local read "Save Array"() -> (w896:string[][])
                n515 = Array Size(array=w896) -> (size(s)=w899:i32[])
                n516 = Array Subset(array=w896, index (row)=0, index (col)=0, length (col)=3) -> (w903:string[][])  [unwired: 1 in]
                n517 = Index Array(array=w899, index=0) -> (element=w897:i32)
                n518 = Reshape Array(w903, w897) -> (w895:string[])
                n519 = Search 1D Array(1D array=w895, element="Length (um):") -> (index of element=w906:i32)  [unwired: 1 in]
                n520 = Equal?(x=w906, y=-1) -> (x = y?=w905:bool)
                n521 = case shown="False" w905 {
                  tunnel: w896 -> [w916 w919]
                  tunnel: w906 -> [w913 _]
                  tunnel: [w912 w919] -> w904
                  frame False {
                    n522 = local read "New: Length"() -> (w909:dbl)
                    n523 = Divide(x=w913, y=3) -> (x/y=w915:dbl)
                    n524 = Format Value(format string="%#g", value (0)=w909) -> (output string=w910:string)  [unwired: 1 in]
                    n525 = To Word Integer(number=w915) -> (16bit integer=w914:i16)
                    n526 = Replace Array Subset(array=w916, new element=w910, index (row)=w914, index (col)=1) -> (w912:string[][])
                  }
                  frame True {
                  }
                }
                n527 = local write "Save Array"(w904) -> ()
              }
              frame #3 {
                n528 = local read "Save Array"() -> (w921:string[][])
                n529 = Array Size(array=w921) -> (size(s)=w926:i32[])
                n530 = Array Subset(array=w921, index (row)=0, index (col)=0, length (col)=3) -> (w922:string[][])  [unwired: 1 in]
                n531 = Index Array(array=w926, index=0) -> (element=w928:i32)
                n532 = Reshape Array(w922, w928) -> (w920:string[])
                n533 = Search 1D Array(1D array=w920, element="Width (um):") -> (index of element=w931:i32)  [unwired: 1 in]
                n534 = Equal?(x=w931, y=-1) -> (x = y?=w930:bool)
                n535 = case shown="False" w930 {
                  tunnel: w931 -> [w939 _]
                  tunnel: w921 -> [w938 w944]
                  tunnel: [w937 w944] -> w929
                  frame False {
                    n536 = local read "New: Width"() -> (w934:dbl)
                    n537 = Divide(x=w939, y=3) -> (x/y=w941:dbl)
                    n538 = To Word Integer(number=w941) -> (16bit integer=w940:i16)
                    n539 = Format Value(format string="%#g", value (0)=w934) -> (output string=w935:string)  [unwired: 1 in]
                    n540 = Replace Array Subset(array=w938, new element=w935, index (row)=w940, index (col)=1) -> (w937:string[][])
                  }
                  frame True {
                  }
                }
                n541 = local write "Save Array"(w929) -> ()
              }
              frame #4 {
                w954 = "Sample Temp (K):"
                n542 = local read "Save Array"() -> (w946:string[][])
                n543 = Array Size(array=w946) -> (size(s)=w951:i32[])
                n544 = Array Subset(array=w946, index (row)=0, index (col)=0, length (col)=3) -> (w947:string[][])  [unwired: 1 in]
                n545 = Index Array(array=w951, index=0) -> (element=w953:i32)
                n546 = Reshape Array(w947, w953) -> (w945:string[])
                n547 = Search 1D Array(1D array=w945, element=w954) -> (index of element=w957:i32)  [unwired: 1 in]
                n548 = Equal?(x=w957, y=-1) -> (x = y?=w956:bool)
                n549 = case shown="True" w956 {
                  tunnel: w946 -> [w966 w980]
                  tunnel: w957 -> [w963 _]
                  tunnel: [w962 w979] -> w955
                  tunnel: w945 -> [_ w982]
                  tunnel: w954 -> [_ w969]
                  frame False {
                    n550 = local read "New: Temp"() -> (w960:dbl)
                    n551 = Divide(x=w963, y=3) -> (x/y=w965:dbl)
                    n552 = Format Value(format string="%#g", value (0)=w960) -> (output string=w959:string)  [unwired: 1 in]
                    n553 = To Word Integer(number=w965) -> (16bit integer=w964:i16)
                    n554 = Replace Array Subset(array=w966, new element=w959, index (row)=w964, index (col)=1) -> (w962:string[][])
                  }
                  frame True {
                    n555 = local read "New: Temp"() -> (w971:dbl)
                    n556 = Search 1D Array(1D array=w982, element="Width (um):") -> (index of element=w976:i32)  [unwired: 1 in]
                    n557 = Divide(x=w976, y=3) -> (x/y=w977:dbl)
                    n558 = To Word Integer(number=w977) -> (16bit integer=w975:i16)
                    n559 = Format Value(format string="%#g", value (0)=w971) -> (output string=w970:string)  [unwired: 1 in]
                    n560 = Build Array(w969, w970) -> (w973:string[])
                    n561 = Increment(x=w975) -> (x+1=w974:i16)
                    n562 = Insert Into Array(array=w980, index (row)=w974, new element=w973) -> (w979:string[][])  [unwired: 1 in]
                  }
                }
                n563 = local write "Save Array"(w955) -> ()
              }
              frame #5 {
                w992 = "Mobility-Sat (cm^2/Vs):"
                n564 = local read "Save Array"() -> (w984:string[][])
                n565 = Array Size(array=w984) -> (size(s)=w989:i32[])
                n566 = Array Subset(array=w984, index (row)=0, index (col)=0, length (col)=3) -> (w985:string[][])  [unwired: 1 in]
                n567 = Index Array(array=w989, index=0) -> (element=w991:i32)
                n568 = Reshape Array(w985, w991) -> (w983:string[])
                n569 = Search 1D Array(1D array=w983, element=w992) -> (index of element=w995:i32)  [unwired: 1 in]
                n570 = Equal?(x=w995, y=-1) -> (x = y?=w994:bool)
                n571 = case shown="True" w994 {
                  tunnel: w984 -> [w1005 w1015]
                  tunnel: w995 -> [w1002 _]
                  tunnel: [w1001 w1014] -> w993
                  tunnel: w983 -> [_ w1012]
                  tunnel: w992 -> [_ w1010]
                  frame False {
                    n572 = local read "Re-Calculated Values Cluster"() -> (w998:T9)
                    n573 = Unbundle By Name(w998) -> ("Mobility-Sat"=w997:dbl)
                    n574 = Divide(x=w1002, y=3) -> (x/y=w1004:dbl)
                    n575 = To Word Integer(number=w1004) -> (16bit integer=w1003:i16)
                    n576 = Format Value(format string="%#g", value (0)=w997) -> (output string=w999:string)  [unwired: 1 in]
                    n577 = Replace Array Subset(array=w1005, new element=w999, index (row)=w1003, index (col)=1) -> (w1001:string[][])
                  }
                  frame True {
                    n578 = local read "Re-Calculated Values Cluster"() -> (w1009:T9)
                    n579 = Unbundle By Name(w1009) -> ("Mobility-Sat"=w1008:dbl)
                    n580 = Search 1D Array(1D array=w1012, element="Mobility (cm^2/Vs):") -> (index of element=w1018:i32)  [unwired: 1 in]
                    n581 = Divide(x=w1018, y=3) -> (x/y=w1019:dbl)
                    n582 = To Word Integer(number=w1019) -> (16bit integer=w1011:i16)
                    n583 = Format Value(format string="%#g", value (0)=w1008) -> (output string=w1013:string)  [unwired: 1 in]
                    n584 = Build Array(w1010, w1013) -> (w1017:string[])
                    n585 = Replace Array Subset(array=w1015, new element=w1017, index (row)=w1011) -> (w1014:string[][])  [unwired: 1 in]
                  }
                }
                n586 = local write "Save Array"(w993) -> ()
              }
              frame #6 {
                w1031 = "Mobility-Lin (cm^2/Vs):"
                n587 = local read "Save Array"() -> (w1022:string[][])
                n588 = Array Size(array=w1022) -> (size(s)=w1028:i32[])
                n589 = Array Subset(array=w1022, index (row)=0, index (col)=0, length (col)=3) -> (w1024:string[][])  [unwired: 1 in]
                n590 = Index Array(array=w1028, index=0) -> (element=w1030:i32)
                n591 = Reshape Array(w1024, w1030) -> (w1023:string[])
                n592 = Search 1D Array(1D array=w1023, element=w1031) -> (index of element=w1034:i32)  [unwired: 1 in]
                n593 = Equal?(x=w1034, y=-1) -> (x = y?=w1033:bool)
                n594 = case shown="True" w1033 {
                  tunnel: w1022 -> [w1044 w1052]
                  tunnel: w1034 -> [w1041 _]
                  tunnel: [w1040 w1051] -> w1032
                  tunnel: w1023 -> [_ w1050]
                  tunnel: w1031 -> [_ w1049]
                  frame False {
                    n595 = local read "Re-Calculated Values Cluster"() -> (w1037:T9)
                    n596 = Unbundle By Name(w1037) -> ("Moblitity-Lin"=w1036:dbl)
                    n597 = Divide(x=w1041, y=3) -> (x/y=w1043:dbl)
                    n598 = To Word Integer(number=w1043) -> (16bit integer=w1042:i16)
                    n599 = Format Value(format string="%#g", value (0)=w1036) -> (output string=w1038:string)  [unwired: 1 in]
                    n600 = Replace Array Subset(array=w1044, new element=w1038, index (row)=w1042, index (col)=1) -> (w1040:string[][])
                  }
                  frame True {
                    n601 = local read "Re-Calculated Values Cluster"() -> (w1048:T9)
                    n602 = Unbundle By Name(w1048) -> ("Moblitity-Lin"=w1047:dbl)
                    n603 = Search 1D Array(1D array=w1050, element="Mobility-Sat (cm^2/Vs):") -> (index of element=w1057:i32)  [unwired: 1 in]
                    n604 = Divide(x=w1057, y=3) -> (x/y=w1058:dbl)
                    n605 = To Word Integer(number=w1058) -> (16bit integer=w1056:i16)
                    n606 = Format Value(format string="%#g", value (0)=w1047) -> (output string=w1061:string)  [unwired: 1 in]
                    n607 = Build Array(w1049, w1061) -> (w1054:string[])
                    n608 = Increment(x=w1056) -> (x+1=w1055:i16)
                    n609 = Insert Into Array(array=w1052, index (row)=w1055, new element=w1054) -> (w1051:string[][])  [unwired: 1 in]
                  }
                }
                n610 = local write "Save Array"(w1032) -> ()
              }
              frame #7 {
                w1071 = "On/Off I-Sat:"
                n611 = local read "Save Array"() -> (w1062:string[][])
                n612 = Array Size(array=w1062) -> (size(s)=w1068:i32[])
                n613 = Array Subset(array=w1062, index (row)=0, index (col)=0, length (col)=3) -> (w1064:string[][])  [unwired: 1 in]
                n614 = Index Array(array=w1068, index=0) -> (element=w1070:i32)
                n615 = Reshape Array(w1064, w1070) -> (w1063:string[])
                n616 = Search 1D Array(1D array=w1063, element=w1071) -> (index of element=w1074:i32)  [unwired: 1 in]
                n617 = Equal?(x=w1074, y=-1) -> (x = y?=w1073:bool)
                n618 = case shown="True" w1073 {
                  tunnel: w1062 -> [w1084 w1093]
                  tunnel: w1074 -> [w1081 _]
                  tunnel: [w1080 w1094] -> w1072
                  tunnel: w1063 -> [_ w1091]
                  tunnel: w1071 -> [_ w1089]
                  frame False {
                    n619 = local read "Calculated Values Cluster"() -> (w1077:T9)
                    n620 = Divide(x=w1081, y=3) -> (x/y=w1083:dbl)
                    n621 = Unbundle By Name(w1077) -> ("On/Off"=w1076:dbl)
                    n622 = To Word Integer(number=w1083) -> (16bit integer=w1082:i16)
                    n623 = Format Value(format string="%#g", value (0)=w1076) -> (output string=w1078:string)  [unwired: 1 in]
                    n624 = Replace Array Subset(array=w1084, new element=w1078, index (row)=w1082, index (col)=1) -> (w1080:string[][])
                  }
                  frame True {
                    n625 = local read "Calculated Values Cluster"() -> (w1088:T9)
                    n626 = Unbundle By Name(w1088) -> ("On/Off"=w1087:dbl)
                    n627 = Search 1D Array(1D array=w1091, element="On/Off Current:") -> (index of element=w1097:i32)  [unwired: 1 in]
                    n628 = Divide(x=w1097, y=3) -> (x/y=w1098:dbl)
                    n629 = To Word Integer(number=w1098) -> (16bit integer=w1090:i16)
                    n630 = Format Value(format string="%#g", value (0)=w1087) -> (output string=w1092:string)  [unwired: 1 in]
                    n631 = Build Array(w1089, w1092) -> (w1096:string[])
                    n632 = Replace Array Subset(array=w1093, new element=w1096, index (row)=w1090) -> (w1094:string[][])  [unwired: 1 in]
                  }
                }
                n633 = local write "Save Array"(w1072) -> ()
              }
              frame #8 {
                w1110 = "Off I-Sat (A):"
                n634 = local read "Save Array"() -> (w1101:string[][])
                n635 = Array Size(array=w1101) -> (size(s)=w1107:i32[])
                n636 = Array Subset(array=w1101, index (row)=0, index (col)=0, length (col)=3) -> (w1103:string[][])  [unwired: 1 in]
                n637 = Index Array(array=w1107, index=0) -> (element=w1109:i32)
                n638 = Reshape Array(w1103, w1109) -> (w1102:string[])
                n639 = Search 1D Array(1D array=w1102, element=w1110) -> (index of element=w1113:i32)  [unwired: 1 in]
                n640 = Equal?(x=w1113, y=-1) -> (x = y?=w1112:bool)
                n641 = case shown="True" w1112 {
                  tunnel: w1101 -> [w1123 w1131]
                  tunnel: w1113 -> [w1120 _]
                  tunnel: [w1119 w1130] -> w1111
                  tunnel: w1102 -> [_ w1129]
                  tunnel: w1110 -> [_ w1128]
                  frame False {
                    # "New Data File"
                    n642 = local read "Calculated Values Cluster"() -> (w1116:T9)
                    n643 = Unbundle By Name(w1116) -> ("Off Current"=w1115:dbl)
                    n644 = Divide(x=w1120, y=3) -> (x/y=w1122:dbl)
                    n645 = Format Value(format string="%#g", value (0)=w1115) -> (output string=w1117:string)  [unwired: 1 in]
                    n646 = To Word Integer(number=w1122) -> (16bit integer=w1121:i16)
                    n647 = Replace Array Subset(array=w1123, new element=w1117, index (row)=w1121, index (col)=1) -> (w1119:string[][])
                  }
                  frame True {
                    # "Old Data File"
                    n648 = local read "Calculated Values Cluster"() -> (w1127:T9)
                    n649 = Unbundle By Name(w1127) -> ("Off Current"=w1126:dbl)
                    n650 = Search 1D Array(1D array=w1129, element="On/Off I-Sat:") -> (index of element=w1136:i32)  [unwired: 1 in]
                    n651 = Divide(x=w1136, y=3) -> (x/y=w1137:dbl)
                    n652 = To Word Integer(number=w1137) -> (16bit integer=w1135:i16)
                    n653 = Format Value(format string="%#g", value (0)=w1126) -> (output string=w1140:string)  [unwired: 1 in]
                    n654 = Build Array(w1128, w1140) -> (w1133:string[])
                    n655 = Increment(x=w1135) -> (x+1=w1134:i16)
                    n656 = Insert Into Array(array=w1131, index (row)=w1134, new element=w1133) -> (w1130:string[][])  [unwired: 1 in]
                  }
                }
                n657 = local write "Save Array"(w1111) -> ()
              }
              frame #9 {
                w1142 = "Vt-Sat (V):"
                n658 = local read "Save Array"() -> (w1143:string[][])
                n659 = Array Size(array=w1143) -> (size(s)=w1148:i32[])
                n660 = Array Subset(array=w1143, index (row)=0, index (col)=0, length (col)=3) -> (w1144:string[][])  [unwired: 1 in]
                n661 = Index Array(array=w1148, index=0) -> (element=w1150:i32)
                n662 = Reshape Array(w1144, w1150) -> (w1141:string[])
                n663 = Search 1D Array(1D array=w1141, element=w1142) -> (index of element=w1153:i32)  [unwired: 1 in]
                n664 = Equal?(x=w1153, y=-1) -> (x = y?=w1152:bool)
                n665 = case shown="True" w1152 {
                  tunnel: w1143 -> [w1162 w1172]
                  tunnel: w1153 -> [w1158 _]
                  tunnel: [w1157 w1171] -> w1151
                  tunnel: w1142 -> [_ w1170]
                  tunnel: w1141 -> [_ w1169]
                  frame False {
                    n666 = local read "Re-Calculated Values Cluster"() -> (w1156:T9)
                    n667 = Unbundle By Name(w1156) -> ("Vt-Sat"=w1155:dbl)
                    n668 = Divide(x=w1158, y=3) -> (x/y=w1161:dbl)
                    n669 = To Word Integer(number=w1161) -> (16bit integer=w1160:i16)
                    n670 = Number To Fractional String(number=w1155) -> (F-format string=w1159:string)  [unwired: 3 in]
                    n671 = Replace Array Subset(array=w1162, new element=w1159, index (row)=w1160, index (col)=1) -> (w1157:string[][])
                  }
                  frame True {
                    n672 = local read "Re-Calculated Values Cluster"() -> (w1166:T9)
                    n673 = Unbundle By Name(w1166) -> ("Vt-Sat"=w1165:dbl)
                    n674 = Search 1D Array(1D array=w1169, element="Threshold V (V):") -> (index of element=w1168:i32)  [unwired: 1 in]
                    n675 = Divide(x=w1168, y=3) -> (x/y=w1175:dbl)
                    n676 = To Word Integer(number=w1175) -> (16bit integer=w1167:i16)
                    n677 = Format Value(format string="%#g", value (0)=w1165) -> (output string=w1178:string)  [unwired: 1 in]
                    n678 = Build Array(w1170, w1178) -> (w1174:string[])
                    n679 = Replace Array Subset(array=w1172, new element=w1174, index (row)=w1167) -> (w1171:string[][])  [unwired: 1 in]
                  }
                }
                n680 = local write "Save Array"(w1151) -> ()
              }
              frame #10 {
                n681 = disable-structure shown="Disabled" {
                  frame Disabled {
                    n682 = local read "Save Array"() -> (w1179:string[][])
                    n683 = Array Size(array=w1179) -> (size(s)=w1185:i32[])
                    n684 = Array Subset(array=w1179, index (row)=0, index (col)=0, length (col)=3) -> (w1181:string[][])  [unwired: 1 in]
                    n685 = Index Array(array=w1185, index=0) -> (element=w1187:i32)
                    n686 = Reshape Array(w1181, w1187) -> (w1180:string[])
                    n687 = Search 1D Array(1D array=w1180, element="VT-Lin (V):") -> (index of element=w1190:i32)  [unwired: 1 in]
                    n688 = Equal?(x=w1190, y=-1) -> (x = y?=w1189:bool)
                    n689 = case shown="False" w1189 {
                      tunnel: w1179 -> [w1199 w1202]
                      tunnel: w1190 -> [w1196 _]
                      tunnel: [w1195 w1202] -> w1188
                      frame False {
                        n690 = Divide(x=w1196, y=3) -> (x/y=w1198:dbl)
                        n691 = To Word Integer(number=w1198) -> (16bit integer=w1197:i16)
                        n692 = Format Value(format string="%#g") -> (output string=w1193:string)  [unwired: 2 in]
                        n693 = Replace Array Subset(array=w1199, new element=w1193, index (row)=w1197, index (col)=1) -> (w1195:string[][])
                      }
                      frame True {
                      }
                    }
                    n694 = local write "Save Array"(w1188) -> ()
                  }
                  frame Enabled {
                  }
                }
              }
              frame #11 {
                w1203 = "STS-Sat (V/decade):"
                n695 = local read "Save Array"() -> (w1205:string[][])
                n696 = Array Size(array=w1205) -> (size(s)=w1210:i32[])
                n697 = Array Subset(array=w1205, index (row)=0, index (col)=0, length (col)=3) -> (w1206:string[][])  [unwired: 1 in]
                n698 = Index Array(array=w1210, index=0) -> (element=w1212:i32)
                n699 = Reshape Array(w1206, w1212) -> (w1204:string[])
                n700 = Search 1D Array(1D array=w1204, element=w1203) -> (index of element=w1215:i32)  [unwired: 1 in]
                n701 = Equal?(x=w1215, y=-1) -> (x = y?=w1214:bool)
                n702 = case shown="True" w1214 {
                  tunnel: w1205 -> [w1225 w1233]
                  tunnel: w1215 -> [w1222 _]
                  tunnel: [w1221 w1234] -> w1213
                  tunnel: w1204 -> [_ w1232]
                  tunnel: w1203 -> [_ w1231]
                  frame False {
                    # "Current Data File"
                    n703 = local read "Re-Calculated Values Cluster"() -> (w1217:T9)
                    n704 = Unbundle By Name(w1217) -> ("STS"=w1218:dbl)
                    n705 = Divide(x=w1222, y=3) -> (x/y=w1224:dbl)
                    n706 = To Word Integer(number=w1224) -> (16bit integer=w1223:i16)
                    n707 = Format Value(format string="%#g", value (0)=w1218) -> (output string=w1219:string)  [unwired: 1 in]
                    n708 = Replace Array Subset(array=w1225, new element=w1219, index (row)=w1223, index (col)=1) -> (w1221:string[][])
                  }
                  frame True {
                    # "Old Data File"
                    n709 = local read "Re-Calculated Values Cluster"() -> (w1228:T9)
                    n710 = Unbundle By Name(w1228) -> ("STS"=w1229:dbl)
                    n711 = Search 1D Array(1D array=w1232, element="S.T.S. (V/decade):") -> (index of element=w1237:i32)  [unwired: 1 in]
                    n712 = Divide(x=w1237, y=3) -> (x/y=w1238:dbl)
                    n713 = To Word Integer(number=w1238) -> (16bit integer=w1230:i16)
                    n714 = Format Value(format string="%#g", value (0)=w1229) -> (output string=w1241:string)  [unwired: 1 in]
                    n715 = Build Array(w1231, w1241) -> (w1236:string[])
                    n716 = Replace Array Subset(array=w1233, new element=w1236, index (row)=w1230) -> (w1234:string[][])  [unwired: 1 in]
                  }
                }
                n717 = local write "Save Array"(w1213) -> ()
              }
              frame #12 {
                w1242 = "Trap Density-VT (Traps/Vcm^2):"
                n718 = local read "Save Array"() -> (w1244:string[][])
                n719 = Array Size(array=w1244) -> (size(s)=w1249:i32[])
                n720 = Array Subset(array=w1244, index (row)=0, index (col)=0, length (col)=3) -> (w1245:string[][])  [unwired: 1 in]
                n721 = Index Array(array=w1249, index=0) -> (element=w1251:i32)
                n722 = Reshape Array(w1245, w1251) -> (w1243:string[])
                n723 = Search 1D Array(1D array=w1243, element=w1242) -> (index of element=w1254:i32)  [unwired: 1 in]
                n724 = Equal?(x=w1254, y=-1) -> (x = y?=w1253:bool)
                n725 = case shown="True" w1253 {
                  tunnel: w1244 -> [w1264 w1271]
                  tunnel: w1254 -> [w1260 _]
                  tunnel: [w1259 w1272] -> w1252
                  tunnel: w1243 -> [_ w1270]
                  tunnel: w1242 -> [_ w1269]
                  frame False {
                    n726 = local read "Re-Calculated Values Cluster"() -> (w1257:T9)
                    n727 = Unbundle By Name(w1257) -> ("Trap Density-VT"=w1256:dbl)
                    n728 = Divide(x=w1260, y=3) -> (x/y=w1263:dbl)
                    n729 = To Word Integer(number=w1263) -> (16bit integer=w1262:i16)
                    n730 = Format Value(format string="%#g", value (0)=w1256) -> (output string=w1261:string)  [unwired: 1 in]
                    n731 = Replace Array Subset(array=w1264, new element=w1261, index (row)=w1262, index (col)=1) -> (w1259:string[][])
                  }
                  frame True {
                    n732 = local read "Re-Calculated Values Cluster"() -> (w1268:T9)
                    n733 = Unbundle By Name(w1268) -> ("Trap Density-VT"=w1267:dbl)
                    n734 = Search 1D Array(1D array=w1270, element="STS-Sat (V/decade):") -> (index of element=w1277:i32)  [unwired: 1 in]
                    n735 = Divide(x=w1277, y=3) -> (x/y=w1276:dbl)
                    n736 = To Word Integer(number=w1276) -> (16bit integer=w1278:i16)
                    n737 = Format Value(format string="%#g", value (0)=w1267) -> (output string=w1273:string)  [unwired: 1 in]
                    n738 = Build Array(w1269, w1273) -> (w1280:string[])
                    n739 = Increment(x=w1278) -> (x+1=w1279:i16)
                    n740 = Insert Into Array(array=w1271, index (row)=w1279, new element=w1280) -> (w1272:string[][])  [unwired: 1 in]
                  }
                }
                n741 = local write "Save Array"(w1252) -> ()
              }
              frame #13 {
                w1282 = "Trap Density-STS (Traps/Vcm^2):"
                n742 = local read "Save Array"() -> (w1284:string[][])
                n743 = Array Size(array=w1284) -> (size(s)=w1289:i32[])
                n744 = Array Subset(array=w1284, index (row)=0, index (col)=0, length (col)=3) -> (w1285:string[][])  [unwired: 1 in]
                n745 = Index Array(array=w1289, index=0) -> (element=w1291:i32)
                n746 = Reshape Array(w1285, w1291) -> (w1283:string[])
                n747 = Search 1D Array(1D array=w1283, element=w1282) -> (index of element=w1294:i32)  [unwired: 1 in]
                n748 = Equal?(x=w1294, y=-1) -> (x = y?=w1293:bool)
                n749 = case shown="True" w1293 {
                  tunnel: w1284 -> [w1304 w1311]
                  tunnel: w1294 -> [w1301 _]
                  tunnel: [w1300 w1312] -> w1292
                  tunnel: w1283 -> [_ w1310]
                  tunnel: w1282 -> [_ w1309]
                  frame False {
                    n750 = local read "Re-Calculated Values Cluster"() -> (w1297:T9)
                    n751 = Unbundle By Name(w1297) -> ("Trap Density-STS"=w1296:dbl)
                    n752 = Divide(x=w1301, y=3) -> (x/y=w1303:dbl)
                    n753 = To Word Integer(number=w1303) -> (16bit integer=w1302:i16)
                    n754 = Format Value(format string="%#g", value (0)=w1296) -> (output string=w1298:string)  [unwired: 1 in]
                    n755 = Replace Array Subset(array=w1304, new element=w1298, index (row)=w1302, index (col)=1) -> (w1300:string[][])
                  }
                  frame True {
                    n756 = local read "Re-Calculated Values Cluster"() -> (w1308:T9)
                    n757 = Unbundle By Name(w1308) -> ("Trap Density-STS"=w1307:dbl)
                    n758 = Search 1D Array(1D array=w1310, element="Trap Density-VT (Traps/Vcm^2):") -> (index of element=w1317:i32)  [unwired: 1 in]
                    n759 = Divide(x=w1317, y=3) -> (x/y=w1318:dbl)
                    n760 = To Word Integer(number=w1318) -> (16bit integer=w1316:i16)
                    n761 = Format Value(format string="%#g", value (0)=w1307) -> (output string=w1321:string)  [unwired: 1 in]
                    n762 = Build Array(w1309, w1321) -> (w1314:string[])
                    n763 = Increment(x=w1316) -> (x+1=w1315:i16)
                    n764 = Insert Into Array(array=w1311, index (row)=w1315, new element=w1314) -> (w1312:string[][])  [unwired: 1 in]
                  }
                }
                n765 = local write "Save Array"(w1292) -> ()
              }
            }
            n766 = local read "New: Temp"() -> (w829:dbl)
            n767 = local read "New: Width"() -> (w830:dbl)
            n768 = local read "New: Length"() -> (w832:dbl)
            n769 = local read "Index"() -> (w831:string)
            n770 = To Single Precision Float(number=w829) -> (single precision float=w846:sgl)
            n771 = Number To Decimal String(number=w846) -> (decimal integer string=w841:string)  [unwired: 1 in]
            n772 = To Single Precision Float(number=w830) -> (single precision float=w845:sgl)
            n773 = To Single Precision Float(number=w832) -> (single precision float=w844:sgl)
            n774 = Strip Path(path=w828) -> (stripped path=w833:path)  [unwired: 1 out]
            n775 = Number To Decimal String(number=w844) -> (decimal integer string=w839:string)  [unwired: 1 in]
            n776 = Number To Decimal String(number=w845) -> (decimal integer string=w838:string)  [unwired: 1 in]
            n777 = Concatenate Strings("_", w841, "K") -> (w843:string)
            n778 = call "Build Text"("Temp"=w843, "Index"=w831, "Length"=w839, "Width"=w838) -> ("Result"=w837:string)  [unwired: 10 in, 1 out]
            n779 = Path To String(path=w833) -> (string=w835:string)
            n780 = Concatenate Strings(w835, "\\", w837) -> (w836:string)
            n781 = String To Path(string=w836) -> (path=w827:path)
          }
          frame #1 {
            n782 = flat-sequence {
              tunnel: w1325 -> [w1327]
              tunnel: w1324 -> [w1326]
              tunnel: [w1326] -> w1323
              tunnel: w1323 -> [w1333]
              tunnel: w1322 -> [w1332]
              frame #0 {
                n783 = Equal?(x=w1327, y=w1326) -> (x = y?=w1328:bool)
                n784 = case shown="False" w1328 {
                  tunnel: w1327 -> [w1331 _]
                  tunnel: w1326 -> [w1330 _]
                  frame False {
                    n785 = Move(source path=w1331, 9:TRUE, 10:w1330) -> ()  [unwired: 2 in, 3 out]
                  }
                  frame True {
                  }
                }
              }
              frame #1 {
                n786 = local write "Transfer File"(w1333) -> ()
                n787 = call-poly <vilib>:"Write To Spreadsheet File.vi"("2D data"=w1332, "file path (dialog if empty)"=w1333) -> ()  [unwired: 6 in, 1 out]
              }
            }
          }
        }
        n788 = Unbundle By Name(w813) -> ("Save Next"=w812:bool)
        n789 = Cluster To Array(cluster=w818) -> (array=w817:bool[])
        n790 = Boolean Array To Number(Boolean array=w817) -> (number=w816:u32)
        n791 = Equal To 0?(x=w816) -> (x = 0?=w815:bool)
        n792 = case shown="True" w815 {
          tunnel: [MegaAwesome_States."Read Data" w825] -> w814
          tunnel: w812 -> [_ w822]
          frame False {
          }
          frame True {
            n793 = Select(t=MegaAwesome_States."No Event", s=w822, f=MegaAwesome_States."Next File") -> (s? t:f=w825:T2)
          }
        }
      }
      frame "Exit" {
        n794 = flat-sequence {
          tunnel: [w1344] -> w1335
          tunnel: [w1344] -> w1334
          frame #0 {
            w1343 = FALSE
            n795 = property on="Next File" class="Bool (strict)"("Value"=w1343) -> (error out=w1338:errorcluster)  [unwired: 2 in, 1 out]
            n796 = property on="Previous File" class="Bool (strict)"(error in=w1338, "Value"=w1343) -> (error out=w1339:errorcluster)  [unwired: 1 in, 1 out]
            n797 = property on="Save" class="Bool (strict)"(error in=w1339, "Value"=w1343) -> (error out=w1340:errorcluster)  [unwired: 1 in, 1 out]
            n798 = property on="Export" class="Bool (strict)"("Value"=w1343) -> ()  [unwired: 2 in, 2 out]
            n799 = property on="Save Next" class="Bool (strict)"(error in=w1340, "Value"=w1343) -> (error out=w1341:errorcluster)  [unwired: 1 in, 1 out]
            n800 = property on="Discard" class="Bool (strict)"(error in=w1341, "Value"=w1343) -> (error out=w1342:errorcluster)  [unwired: 1 in, 1 out]
            n801 = property on="Save Lines" class="Bool (strict)"(error in=w1342, "Value"=w1343) -> ()  [unwired: 1 in, 2 out]
            n802 = property on="Close" class="Bool (strict)"("Value"=w1343) -> ()  [unwired: 2 in, 2 out]
            n803 = property on="Disable Flag" class="Bool (strict)"("Value"=w1343) -> ()  [unwired: 2 in, 2 out]
            n804 = call "IMAQ Dispose"("All Images? (No)"=TRUE) -> ()  [unwired: 5 in, 1 out]
          }
          frame #1 {
            w1344 = MegaAwesome_States."Exit"
          }
        }
      }
      frame "Save Lines" {
        n805 = Build Path(base path=w1346, name or relative path="ROI") -> (appended path=w1349:path)
        n806 = call <vilib>:"Check if File or Folder Exists.vi"("path"=w1349) -> ("file or folder exists?"=w1347:bool, "dup path"=w1350:path)  [unwired: 8 in, 1 out]
        n807 = case shown="False" w1347 {
          tunnel: w1350 -> [w1358 w1359]
          tunnel: [w1357 w1359] -> w1354
          frame False {
            n808 = Create Folder(path (use dialog)=w1358) -> (created path=w1357:path)  [unwired: 2 in, 2 out]
          }
          frame True {
          }
        }
        n809 = local read "Index"() -> (w1345:string)
        n810 = property on="Image Out" class="ImageControl"() -> ("ROI"=w1351:T17)  [unwired: 2 in, 2 out]
        n811 = Build Path(base path=w1354, name or relative path=w1345) -> (appended path=w1353:path)
        n812 = Flatten To String(anything=w1351) -> (data string=w1352:string)  [unwired: 3 in, 2 out]
        n813 = Write to Text File(file (use dialog)=w1353, text=w1352) -> ()  [unwired: 2 in, 3 out]
      }
      frame "Export" {
        n814 = flat-sequence {
          tunnel: ["Independant Variable:"] -> w1360
          tunnel: w1361 -> [w1416]
          tunnel: w1360 -> [w1415]
          frame #0 {
            n815 = stacked-sequence {
              tunnel: "Independant Variable:" -> [w1365 w1370 w1375 w1380 w1385 w1390 w1395 w1400 w1405 w1410]
              frame #0 {
                n816 = Equal?(x=w1365, y="Length (um):") -> (x = y?=w1366:bool)
                n817 = case shown="True" w1366 {
                  frame False {
                  }
                  frame True {
                    n818 = local write "X Axis Display Type"("1") -> ()
                    n819 = local write "Opj X Axis"("2") -> ()
                  }
                }
              }
              frame #1 {
                n820 = Equal?(x=w1370, y="Sample Temp (K):") -> (x = y?=w1371:bool)
                n821 = case shown="True" w1371 {
                  frame False {
                  }
                  frame True {
                    n822 = local write "X Axis Display Type"("1") -> ()
                    n823 = local write "Opj X Axis"("1") -> ()
                  }
                }
              }
              frame #2 {
                n824 = Equal?(x=w1375, y="Mobility-Sat (cm^2/Vs):") -> (x = y?=w1376:bool)
                n825 = case shown="True" w1376 {
                  frame False {
                  }
                  frame True {
                    n826 = local write "X Axis Display Type"("2") -> ()
                    n827 = local write "Opj X Axis"("2") -> ()
                  }
                }
              }
              frame #3 {
                n828 = Equal?(x=w1380, y="Mobility-Lin (cm^2/Vs):") -> (x = y?=w1381:bool)
                n829 = case shown="True" w1381 {
                  frame False {
                  }
                  frame True {
                    n830 = local write "X Axis Display Type"("2") -> ()
                    n831 = local write "Opj X Axis"("2") -> ()
                  }
                }
              }
              frame #4 {
                n832 = Equal?(x=w1385, y="On/Off I-Sat:") -> (x = y?=w1386:bool)
                n833 = case shown="True" w1386 {
                  frame False {
                  }
                  frame True {
                    n834 = local write "X Axis Display Type"("2") -> ()
                    n835 = local write "Opj X Axis"("2") -> ()
                  }
                }
              }
              frame #5 {
                n836 = Equal?(x=w1390, y="Off I-Sat (A):") -> (x = y?=w1391:bool)
                n837 = case shown="True" w1391 {
                  frame False {
                  }
                  frame True {
                    n838 = local write "X Axis Display Type"("2") -> ()
                    n839 = local write "Opj X Axis"("2") -> ()
                  }
                }
              }
              frame #6 {
                n840 = Equal?(x=w1395, y="Vt-Sat (V):") -> (x = y?=w1396:bool)
                n841 = case shown="True" w1396 {
                  frame False {
                  }
                  frame True {
                    n842 = local write "X Axis Display Type"("1") -> ()
                    n843 = local write "Opj X Axis"("1") -> ()
                  }
                }
              }
              frame #7 {
                n844 = Equal?(x=w1400, y="STS-Sat (V/decade):") -> (x = y?=w1401:bool)
                n845 = case shown="True" w1401 {
                  frame False {
                  }
                  frame True {
                    n846 = local write "X Axis Display Type"("1") -> ()
                    n847 = local write "Opj X Axis"("1") -> ()
                  }
                }
              }
              frame #8 {
                n848 = Equal?(x=w1405, y="Trap Density-VT (Traps/Vcm^2):") -> (x = y?=w1406:bool)
                n849 = case shown="True" w1406 {
                  frame False {
                  }
                  frame True {
                    n850 = local write "X Axis Display Type"("2") -> ()
                    n851 = local write "Opj X Axis"("2") -> ()
                  }
                }
              }
              frame #9 {
                n852 = Equal?(x=w1410, y="Trap Density-STS (Traps/Vcm^2):") -> (x = y?=w1411:bool)
                n853 = case shown="True" w1411 {
                  frame False {
                  }
                  frame True {
                    n854 = local write "X Axis Display Type"("2") -> ()
                    n855 = local write "Opj X Axis"("2") -> ()
                  }
                }
              }
            }
          }
          frame #1 {
            n856 = local read "Transfer Folder"() -> (w1420:path)
            n857 = Build Path(base path=w1420, name or relative path="Stats") -> (appended path=w1421:path)
            n858 = call <vilib>:"Check if File or Folder Exists.vi"("path"=w1421) -> ("file or folder exists?"=w1435:bool, "dup path"=w1434:path)  [unwired: 8 in, 1 out]
            n859 = call <userlib>:"OA_ConnectToOrigin.vi"() -> ("error out"=w1432:errorcluster, "Origin.IOApplication"=w1433:refnum<k7>)  [unwired: 8 in]
            n860 = case shown="False" w1435 {
              tunnel: w1434 -> [w1608 w1609]
              tunnel: [w1607 w1609] -> w1419
              frame False {
                n861 = Create Folder(path (use dialog)=w1608) -> (created path=w1607:path)  [unwired: 2 in, 2 out]
              }
              frame True {
              }
            }
            n862 = call "File Dialog"("start path"=w1421) -> ("selected path"=w1423:path)  [unwired: 11 in, 3 out]
            n863 = call <userlib>:"OA_Load.vi"("error in (no error)"=w1432, "Path"=w1416, "Origin.IOApplication"=w1433) -> ("error out"=w1430:errorcluster, "Origin.IOApplication"=w1431:refnum<k7>)  [unwired: 1 out]
            n864 = call "OAExecute.vi"("script"="document -m 3;", "Error IO"=w1430, "Origin.IOApplication"=w1431) -> ("Error IO Out"=w1428:errorcluster, "Origin.IOApplication"=w1429:refnum<k7>)  [unwired: 1 in, 1 out]
            n865 = stacked-sequence {
              tunnel: w1420 -> [w1446 w1476 w1488 w1510 w1530 w1551 w1572 w1595]
              tunnel: w1419 -> [w1447 w1475 w1489 w1509 w1531 w1552 w1573 w1596]
              tunnel: w1429 -> [w1449 w1473 w1491 w1512 w1533 w1554 w1575 w1598]
              tunnel: w1428 -> [w1448 w1474 w1490 w1511 w1532 w1553 w1574 w1597]
              tunnel: [_ _ _ _ _ _ _ w1593] -> w1418
              tunnel: [_ _ _ _ _ _ _ w1594] -> w1417
              tunnel: w1415 -> [w1445 w1466 w1487 w1508 w1529 w1550 w1571 w1592]
              frame #0 {
                n866 = local read "X Axis Display Type"() -> (w1437:string)
                n867 = local read "Opj X Axis"() -> (w1442:string)
                n868 = Concatenate Strings("window -a MOBLGraph;\nlayer.x.type=", w1442, "; layer.x.label.numFormat = ", w1437, "; Y3 = 1; X3 = 1;", "window -a MOBLTable;\nwindow -s TV;") -> (w1440:string)
                n869 = call "Param_Analysis_7_24b_JW.vi"("Independant Variable"=w1445, "error in (no error)"=w1448, "Data Folder"=w1446, "Parameter String"="Mobility-Lin (cm^2/Vs):", "Parameter Name"="Mobility-Lin", "Stats Folder"=w1447) -> ("error out"=w1451:errorcluster, "Output Array"=w1453:string[][], "Variables"=w1444:T27)  [unwired: 2 in, 1 out]
                n870 = call "Origin_Export_7_27a_JW.vi"("Input Conditions"=w1444, "Analysis Array"=w1453, "error in (no error)"=w1451, "Parameter Worksheet Name"="[MOBLTable]Mobilities", "Parameter Folder Script"="pe_cd \"Mobility-Lin\";", "Origin.IOApplication"=w1449) -> ("error out"=w1450:errorcluster, "reference out"=w1452:refnum<k7>)  [unwired: 3 in, 1 out]
                n871 = call "OAExecute.vi"("script"=w1440, "Error IO"=w1450, "Origin.IOApplication"=w1452) -> ()  [unwired: 1 in, 3 out]
              }
              frame #1 {
                n872 = local read "X Axis Display Type"() -> (w1458:string)
                n873 = local read "Opj X Axis"() -> (w1463:string)
                n874 = Concatenate Strings("window -a MOBSGraph;\nlayer.x.type=", w1463, "; layer.x.label.numFormat = ", w1458, "; Y3 = 1; X3 = 1;", "window -a MOBSTable;\nwindow -s TV;") -> (w1461:string)
                n875 = call "Param_Analysis_7_24b_JW.vi"("Independant Variable"=w1466, "error in (no error)"=w1474, "Data Folder"=w1476, "Parameter String"="Mobility-Sat (cm^2/Vs):", "Parameter Name"="Mobility-Sat", "Stats Folder"=w1475) -> ("error out"=w1469:errorcluster, "Output Array"=w1467:string[][], "Variables"=w1465:T27)  [unwired: 2 in, 1 out]
                n876 = call "Origin_Export_7_27a_JW.vi"("Input Conditions"=w1465, "Analysis Array"=w1467, "error in (no error)"=w1469, "Parameter Worksheet Name"="[MOBSTable]Mobilities", "Parameter Folder Script"="pe_cd \"Mobility-Sat\";", "Origin.IOApplication"=w1473) -> ("error out"=w1468:errorcluster, "reference out"=w1470:refnum<k7>)  [unwired: 3 in, 1 out]
                n877 = call "OAExecute.vi"("script"=w1461, "Error IO"=w1468, "Origin.IOApplication"=w1470) -> ()  [unwired: 1 in, 3 out]
              }
              frame #2 {
                n878 = local read "X Axis Display Type"() -> (w1479:string)
                n879 = local read "Opj X Axis"() -> (w1484:string)
                n880 = Concatenate Strings("window -a NSTSGraph;\nlayer.x.type=", w1484, "; layer.x.label.numFormat = ", w1479, "; Y3 = 1; X3 = 1;", "window -a NSTSTable;\nwindow -s TV;") -> (w1482:string)
                n881 = call "Param_Analysis_7_24b_JW.vi"("Independant Variable"=w1487, "error in (no error)"=w1490, "Data Folder"=w1488, "Parameter String"="Trap Density-STS (Traps/Vcm^2):", "Parameter Name"="Trap Density-STS", "Stats Folder"=w1489) -> ("error out"=w1494:errorcluster, "Output Array"=w1492:string[][], "Variables"=w1486:T27)  [unwired: 2 in, 1 out]
                n882 = call "Origin_Export_7_27a_JW.vi"("Input Conditions"=w1486, "Analysis Array"=w1492, "error in (no error)"=w1494, "Parameter Worksheet Name"="[NSTSTable]Trap Densities", "Parameter Folder Script"="pe_cd \"N-STS\";", "Origin.IOApplication"=w1491) -> ("error out"=w1493:errorcluster, "reference out"=w1495:refnum<k7>)  [unwired: 3 in, 1 out]
                n883 = call "OAExecute.vi"("script"=w1482, "Error IO"=w1493, "Origin.IOApplication"=w1495) -> ()  [unwired: 1 in, 3 out]
              }
              frame #3 {
                n884 = local read "X Axis Display Type"() -> (w1500:string)
                n885 = local read "Opj X Axis"() -> (w1505:string)
                n886 = call "Param_Analysis_7_24b_JW.vi"("Independant Variable"=w1508, "error in (no error)"=w1511, "Data Folder"=w1510, "Parameter String"="Trap Density-VT (Traps/Vcm^2):", "Parameter Name"="Trap Density-Vt", "Stats Folder"=w1509) -> ("error out"=w1515:errorcluster, "Output Array"=w1513:string[][], "Variables"=w1507:T27)  [unwired: 2 in, 1 out]
                n887 = Concatenate Strings("window -a NVtGraph;\nlayer.x.type=", w1505, "; layer.x.label.numFormat = ", w1500, "; Y3 = 1; X3 = 1;", "window -a NVtTable;\nwindow -s TV;") -> (w1503:string)
                n888 = call "Origin_Export_7_27a_JW.vi"("Input Conditions"=w1507, "Analysis Array"=w1513, "error in (no error)"=w1515, "Parameter Worksheet Name"="[NVTTable]Trap Densities", "Parameter Folder Script"="pe_cd \"N-Vt\";", "Origin.IOApplication"=w1512) -> ("error out"=w1514:errorcluster, "reference out"=w1516:refnum<k7>)  [unwired: 3 in, 1 out]
                n889 = call "OAExecute.vi"("script"=w1503, "Error IO"=w1514, "Origin.IOApplication"=w1516) -> ()  [unwired: 1 in, 3 out]
              }
              frame #4 {
                n890 = local read "X Axis Display Type"() -> (w1521:string)
                n891 = local read "Opj X Axis"() -> (w1526:string)
                n892 = Concatenate Strings("window -a OffIGraph;\nlayer.x.type=", w1526, "; layer.x.label.numFormat = ", w1521, "; Y3 = 1; X3 = 1;", "window -a OffITable;\nwindow -s TV;") -> (w1524:string)
                n893 = call "Param_Analysis_7_24b_JW.vi"("Independant Variable"=w1529, "error in (no error)"=w1532, "Data Folder"=w1530, "Parameter String"="Off I-Sat (A):", "Parameter Name"="Off I-Sat", "Stats Folder"=w1531) -> ("error out"=w1536:errorcluster, "Output Array"=w1534:string[][], "Variables"=w1528:T27)  [unwired: 2 in, 1 out]
                n894 = call "Origin_Export_7_27a_JW.vi"("Input Conditions"=w1528, "Analysis Array"=w1534, "error in (no error)"=w1536, "Parameter Worksheet Name"="[OffItable]OffCurrents", "Parameter Folder Script"="pe_cd \"OffI-Sat\";", "Origin.IOApplication"=w1533) -> ("error out"=w1535:errorcluster, "reference out"=w1537:refnum<k7>)  [unwired: 3 in, 1 out]
                n895 = call "OAExecute.vi"("script"=w1524, "Error IO"=w1535, "Origin.IOApplication"=w1537) -> ()  [unwired: 1 in, 3 out]
              }
              frame #5 {
                n896 = local read "X Axis Display Type"() -> (w1542:string)
                n897 = local read "Opj X Axis"() -> (w1547:string)
                n898 = Concatenate Strings("window -a OnOffGraph;\nlayer.x.type=", w1547, "; layer.x.label.numFormat = ", w1542, "; Y3 = 1; X3 = 1;", "window -a OnOffTable;\nwindow -s TV;") -> (w1545:string)
                n899 = call "Param_Analysis_7_24b_JW.vi"("Independant Variable"=w1550, "error in (no error)"=w1553, "Data Folder"=w1551, "Parameter String"="On/Off I-Sat:", "Parameter Name"="OnOff Ratio", "Stats Folder"=w1552) -> ("error out"=w1557:errorcluster, "Output Array"=w1555:string[][], "Variables"=w1549:T27)  [unwired: 2 in, 1 out]
                n900 = call "Origin_Export_7_27a_JW.vi"("Input Conditions"=w1549, "Analysis Array"=w1555, "error in (no error)"=w1557, "Parameter Worksheet Name"="[OnOffTable]On/Off Ratios", "Parameter Folder Script"="pe_cd \"OnOff-Ratio\";", "Origin.IOApplication"=w1554) -> ("error out"=w1556:errorcluster, "reference out"=w1558:refnum<k7>)  [unwired: 3 in, 1 out]
                n901 = call "OAExecute.vi"("script"=w1545, "Error IO"=w1556, "Origin.IOApplication"=w1558) -> ()  [unwired: 1 in, 3 out]
              }
              frame #6 {
                n902 = local read "X Axis Display Type"() -> (w1563:string)
                n903 = local read "Opj X Axis"() -> (w1568:string)
                n904 = call "Param_Analysis_7_24b_JW.vi"("Independant Variable"=w1571, "error in (no error)"=w1574, "Data Folder"=w1572, "Parameter String"="STS-Sat (V/decade):", "Parameter Name"="STS-Sat", "Stats Folder"=w1573) -> ("error out"=w1578:errorcluster, "Output Array"=w1576:string[][], "Variables"=w1570:T27)  [unwired: 2 in, 1 out]
                n905 = Concatenate Strings("window -a SGraph;\nlayer.x.type=", w1568, "; layer.x.label.numFormat = ", w1563, "; Y3 = 1; X3 = 1;", "window -a STable;\nwindow -s TV;") -> (w1566:string)
                n906 = call "Origin_Export_7_27a_JW.vi"("Input Conditions"=w1570, "Analysis Array"=w1576, "error in (no error)"=w1578, "Parameter Worksheet Name"="[STable]Threshold Swing", "Parameter Folder Script"="pe_cd \"STS-Sat\";", "Origin.IOApplication"=w1575) -> ("error out"=w1577:errorcluster, "reference out"=w1579:refnum<k7>)  [unwired: 3 in, 1 out]
                n907 = call "OAExecute.vi"("script"=w1566, "Error IO"=w1577, "Origin.IOApplication"=w1579) -> ()  [unwired: 1 in, 3 out]
              }
              frame #7 {
                n908 = local read "X Axis Display Type"() -> (w1584:string)
                n909 = local read "Opj X Axis"() -> (w1589:string)
                n910 = Concatenate Strings("window -a VtGraph;\nlayer.x.type=", w1589, "; layer.x.label.numFormat = ", w1584, "; Y3 = 1; X3 = 1;", "window -a VtTable;\nwindow -s TV;") -> (w1587:string)
                n911 = call "Param_Analysis_7_24b_JW.vi"("Independant Variable"=w1592, "error in (no error)"=w1597, "Data Folder"=w1595, "Parameter String"="Vt-Sat (V):", "Parameter Name"="Vt-Sat", "Stats Folder"=w1596) -> ("error out"=w1601:errorcluster, "Output Array"=w1599:string[][], "Variables"=w1591:T27)  [unwired: 2 in, 1 out]
                n912 = call "Origin_Export_7_27a_JW.vi"("Input Conditions"=w1591, "Analysis Array"=w1599, "error in (no error)"=w1601, "Parameter Worksheet Name"="[VtTable]Threshold Voltages", "Parameter Folder Script"="pe_cd \"Vt-Sat\";", "Origin.IOApplication"=w1598) -> ("error out"=w1600:errorcluster, "reference out"=w1602:refnum<k7>)  [unwired: 3 in, 1 out]
                n913 = call "OAExecute.vi"("script"=w1587, "Error IO"=w1600, "Origin.IOApplication"=w1602) -> ("Error IO Out"=w1593:errorcluster, "Origin.IOApplication"=w1594:refnum<k7>)  [unwired: 1 in, 1 out]
              }
            }
            n914 = Path To String(path=w1423) -> (string=w1422:string)
            n915 = call "OAExecute.vi"("script"="pe_cd /; ", "Error IO"=w1418, "Origin.IOApplication"=w1417) -> ("Error IO Out"=w1424:errorcluster, "Origin.IOApplication"=w1425:refnum<k7>)  [unwired: 1 in, 1 out]
            n916 = call <userlib>:"OASaveProject.vi"("path"=w1422, "Error IO"=w1424, "Origin.IOApplication"=w1425) -> ()  [unwired: 3 out]
          }
        }
      }
    }
    "Current State" <- w16
    "Folder Index" <- w23
    n917 = Wait (ms)(milliseconds to wait=u32 50) -> ()  [unwired: 1 out]
    n918 = Equal?(x=w13, y=MegaAwesome_States."Exit") -> (x = y?=w15:bool)
  }
  n919 = call "Close LabView?"("Enable"=w2) -> ("OK"=w1:bool)  [unwired: 17 in, 1 out]
  n920 = Quit LabVIEW(quit? (T)=w1) -> ()
